vi "rio 9030.vi"() -> ()   [LabVIEW 2015]
uses:
  rio_Global.vi
  <vilib>/rvi/interface/nirviMethod/nirviMethod.xnode
  <vilib>/FPGAPlugInAG/Dynamic/niLvFpga_ReadFifo_Dynamic.vi
  <vilib>/rvi/errors/niLvFpgaMergeErrorWithErrorCode.vi
  <vilib>/FPGAPlugInAG/Dynamic/niLvFpga_Abort_Dynamic.vi
  <vilib>/FPGAPlugInAG/Dynamic/niLvFpga_Run_Dynamic.vi
  <vilib>/Analysis/Matrix/NI_Matrix.lvlib
  <vilib>/Analysis/Matrix/Numeric/Multiply/Multiply - RM,RM.vi
  <vilib>/Analysis/Matrix/Numeric/Subtract/Subtract - RM,RM.vi
  <vilib>/Analysis/Matrix/Numeric/Conversions/Array To Matrix - RA.vi
  <vilib>/Analysis/Matrix/Numeric/Add/Add - RM,RM.vi
  <vilib>/Analysis/NI_AALBase.lvlib
  <vilib>/rvi/interface/nirviReadWriteControl/nirviReadWriteControl.xnode
  <vilib>/Utility/error.llb/Error Cluster From Error Code.vi
  <vilib>/rvi/interface/Simulation/niFpgaSimulationCallBeginRW.vi
  <vilib>/rvi/errors/niLvFpgaAdjustHostInterfaceError.vi
  NiFpgaLv.dll
  <vilib>/rvi/interface/nirviOpenFPGA/nirviOpenFPGA.xnode
  FPGA Bitfiles/autonomous_FPGATarget4_fpga1_rudp+OsNkSQ.lvbitx
  samsung/fpga 1.vi
  <vilib>/Analysis/Matrix/Numeric/Multiply/Multiply - R,RM.vi
  <vilib>/Analysis/baseanly.llb/Real Inverse Matrix.vi
  <vilib>/Analysis/Matrix/Numeric/Conversions/Matrix To Array - RM.vi
  <vilib>/Analysis/Matrix/Numeric/Conversions/Array To Matrix - RA2.vi
panel:
  out "XY Graph":cluster{"Y":dbl[], "Y":dbl[]}[](graph)=[{"Y"=[1.82421875, 1.8301353427767753, 1.835194070339203, 1.8394013252854347, 1.8427635002136231, 1.84528698772192, 1.8469781804084777, 1.8478434708714486, 1.8478892517089844, 1.8471219155192375, 1.84554785490036, 1.8431734624505043, 1.8400051307678222, 1.8360492524504661, 1.8313122200965881, 1.8258004263043404, 1.819520263671875, 1.8124781247973443, 1.8046804022789003, 1.796133488714695, 1.7868437767028809, 1.77681765884161, 1.7660615277290344, 1.7545817759633064, 1.742384796142578, 1.7294769808650017, 1.7158647227287291, 1.701554414331913, 1.686552448272705, 1.6708652171492577, 1.654499113559723, 1.637460530102253, 1.619755859375, 1.6013914939761162, 1.5823738265037537, 1.5627092495560646, 1.5424041557312012, 1.5214649376273155, 1.4998979878425598, 1.4777096989750862, 1.4549064636230469, 1.431494674384594, 1.4074807238578795, 1.3828710046410562, 1.3576719093322753, 1.3318898305296898, 1.3055311608314515, 1.2786022928357124, 1.251109619140625, 1.2230595323443412], "Y"=[0.0, 0.5, 1.0, 1.5, 2.0, 2.5, 3.0, 3.5, 4.0, 4.5, 5.0, 5.5, 6.0, 6.5, 7.0, 7.5, 8.0, 8.5, 9.0, 9.5, 10.0, 10.5, 11.0, 11.5, 12.0, 12.5, 13.0, 13.5, 14.0, 14.5, 15.0, 15.5, 16.0, 16.5, 17.0, 17.5, 18.0, 18.5, 19.0, 19.5, 20.0, 20.5, 21.0, 21.5, 22.0, 22.5, 23.0, 23.5, 24.0, 24.5]}, {"Y"=[-1.22265625, -1.2167396572232247, -1.211680929660797, -1.2074736747145653, -1.2041114997863769, -1.20158801227808, -1.1998968195915223, -1.1990315291285514, -1.1989857482910156, -1.1997530844807625, -1.20132714509964, -1.2037015375494957, -1.2068698692321778, -1.2108257475495339, -1.2155627799034119, -1.2210745736956596, -1.227354736328125, -1.2343968752026557, -1.2421945977210997, -1.250741511285305, -1.2600312232971191, -1.27005734115839, -1.2808134722709656, -1.2922932240366936, -1.304490203857422, -1.3173980191349983, -1.3310102772712709, -1.345320585668087, -1.360322551727295, -1.3760097828507423, -1.392375886440277, -1.409414469897747, -1.427119140625, -1.4454835060238838, -1.4645011734962463, -1.4841657504439354, -1.5044708442687988, -1.5254100623726845, -1.5469770121574402, -1.5691653010249138, -1.5919685363769531, -1.615380325615406, -1.6393942761421205, -1.6640039953589438, -1.6892030906677247, -1.7149851694703102, -1.7413438391685485, -1.7682727071642876, -1.795765380859375, -1.8238154676556588, -1.8524165749549866, -1.8815623101592065, -1.911246280670166, -1.9414620938897134, -1.972203357219696, -2.003463678061962, -2.0352366638183597, -2.0675159218907355, -2.1002950596809384, -2.1335676845908162, -2.167327404022217, -2.2015678253769875, -2.2362825560569766, -2.2714652034640315, -2.307109375, -2.3432086780667305, -2.3797567200660703, -2.4167471083998677, -2.4541734504699706, -2.4920293536782263, -2.530308425426483, -2.5690042731165885, -2.6081105041503907, -2.647620725929737, -2.687528545856476, -2.7278275713324547, -2.7685114097595216, -2.809573668539524, -2.8510079550743104, -2.892807876765728, -2.934967041015625, -2.977479055225849, -3.020337526798248, -3.0635360631346704, -3.107068271636963, -3.150927759706974, -3.1951081347465515, -3.2396030041575434, -3.284405975341797, -3.3295106557011604, -3.3749106526374817, -3.4205995735526087, -3.466571025848389, -3.51281861692667, -3.5593359541893004], "Y"=[0.0, 0.5, 1.0, 1.5, 2.0, 2.5, 3.0, 3.5, 4.0, 4.5, 5.0, 5.5, 6.0, 6.5, 7.0, 7.5, 8.0, 8.5, 9.0, 9.5, 10.0, 10.5, 11.0, 11.5, 12.0, 12.5, 13.0, 13.5, 14.0, 14.5, 15.0, 15.5, 16.0, 16.5, 17.0, 17.5, 18.0, 18.5, 19.0, 19.5, 20.0, 20.5, 21.0, 21.5, 22.0, 22.5, 23.0, 23.5, 24.0, 24.5, 25.0, 25.5, 26.0, 26.5, 27.0, 27.5, 28.0, 28.5, 29.0, 29.5, 30.0, 30.5, 31.0, 31.5, 32.0, 32.5, 33.0, 33.5, 34.0, 34.5, 35.0, 35.5, 36.0, 36.5, 37.0, 37.5, 38.0, 38.5, 39.0, 39.5, 40.0, 40.5, 41.0, 41.5, 42.0, 42.5, 43.0, 43.5, 44.0, 44.5, 45.0, 45.5, 46.0, 46.5, 47.0]}, {"Y"=[-0.94, 0.94, 0.94, -0.94, -0.94], "Y"=[-3.2, -3.2, 1.5, 1.5, -3.2]}, {"Y"=[1.984375, 1.978057861328125, 1.9718017578125, 1.965606689453125, 1.95947265625], "Y"=[0.0, 0.5, 1.0, 1.5, 2.0]}, {"Y"=[-5.28125, -5.267578125, -5.25390625, -5.240234375, -5.2265625], "Y"=[0.0, 0.5, 1.0, 1.5, 2.0]}]
  out "x_view":dbl[](array[numeric])=[0.0, 0.5, 1.0, 1.5, 2.0, 2.5, 3.0, 3.5, 4.0, 4.5, 5.0, 5.5, 6.0, 6.5, 7.0, 7.5, 8.0, 8.5, 9.0, 9.5, 10.0, 10.5, 11.0, 11.5, 12.0, 12.5, 13.0, 13.5, 14.0, 14.5, 15.0, 15.5, 16.0, 16.5, 17.0, 17.5, 18.0, 18.5, 19.0, 19.5, 20.0, 20.5, 21.0, 21.5, 22.0, 22.5, 23.0, 23.5, 24.0, 24.5, 25.0, 25.5, 26.0, 26.5, 27.0, 27.5, 28.0, 28.5, 29.0, 29.5, 30.0, 30.5, 31.0, 31.5, 32.0, 32.5, 33.0, 33.5, 34.0, 34.5, 35.0, 35.5, 36.0, 36.5, 37.0, 37.5, 38.0, 38.5, 39.0, 39.5, 40.0, 40.5, 41.0, 41.5, 42.0, 42.5, 43.0, 43.5, 44.0, 44.5, 45.0, 45.5, 46.0, 46.5, 47.0, 47.5, 48.0, 48.5, 49.0, 49.5, 50.0, 50.5, 51.0, 51.5, 52.0, 52.5, 53.0, 53.5, 54.0, 54.5, 55.0, 55.5, 56.0, 56.5, 57.0, 57.5, 58.0, 58.5, 59.0, 59.5, 60.0, 60.5, 61.0, 61.5, 62.0, 62.5, 63.0, 63.5, 64.0, 64.5, 65.0, 65.5, 66.0, 66.5, 67.0, 67.5, 68.0, 68.5, 69.0, 69.5, 70.0, 70.5, 71.0, 71.5, 72.0, 72.5, 73.0, 73.5, 74.0, 74.5, 75.0, 75.5, 76.0, 76.5, 77.0, 77.5, 78.0, 78.5, 79.0, 79.5, 80.0, 80.5, 81.0, 81.5, 82.0, 82.5, 83.0, 83.5, 84.0, 84.5, 85.0, 85.5, 86.0, 86.5, 87.0, 87.5, 88.0, 88.5, 89.0, 89.5, 90.0, 90.5, 91.0, 91.5, 92.0, 92.5, 93.0, 93.5, 94.0, 94.5, 95.0, 95.5, 96.0, 96.5, 97.0, 97.5, 98.0, 98.5, 99.0, 99.5, 100.0, 100.5, 101.0, 101.5, 102.0, 102.5, 103.0, 103.5, 104.0, 104.5, 105.0, 105.5, 106.0, 106.5, 107.0, 107.5, 108.0, 108.5, 109.0, 109.5, 110.0, 110.5, 111.0, 111.5, 112.0, 112.5, 113.0, 113.5, 114.0, 114.5, 115.0, 115.5, 116.0, 116.5, 117.0, 117.5, 118.0, 118.5, 119.0, 119.5, 120.0, 120.5, 121.0, 121.5, 122.0, 122.5, 123.0, 123.5, 124.0, 124.5, 125.0, 125.5, 126.0, 126.5, 127.0, 127.5, 128.0]
  in  "rate limit":dbl=0.006 format="%#_13g"
  in  "Manual Steering torque":dbl(slide) min=-0.3 max=0.3 step=0.01 scale=-0.3..0.3
  out "T init":i32
  out "T out":i32
  out "PWM GAS":dbl=1000.0 min=1000.0 max=2000.0 step=1.0
  out "FPGA":refnum<k20>
  out "Mobileye_time 50":u32
  out "H_GPS":dbl
  out "vgain":dbl=1.0
  out "vcount":u64=1
  out "hbias":dbl
  out "hcount":u64=1
  out "get heading":bool
  out "get position":bool
  out "heading error":dbl
  out "h_gps":dbl
  out "rt":dbl
  out "pos error":dbl
  out "POS init":bool
  out "Heading":dbl
  out "pos":dbl[](array[numeric])
  in  "GPS init":bool=TRUE
  out "pos_gps":dbl[](array[numeric]) format="%#_19f"
  out "dt":dbl
  out "Pos_time 10":i32
  out "Ref_steer_planner":dbl
  out "Ref_vel_planner":dbl
  out "map":i32=2
  out "ecef ref":dbl[](array[numeric])
  in  "Velocity input":bool
  in  "manual Speed":dbl
  in  "Steer input":bool=TRUE
  out "Run":bool
  out "Auto":bool
  out "E - STOP":bool
  out "Con_time 10":i32
  out "VS_CAN":dbl
  out "CAN_time 10":u32
  out "gps1":refnum<visa-resource-name>
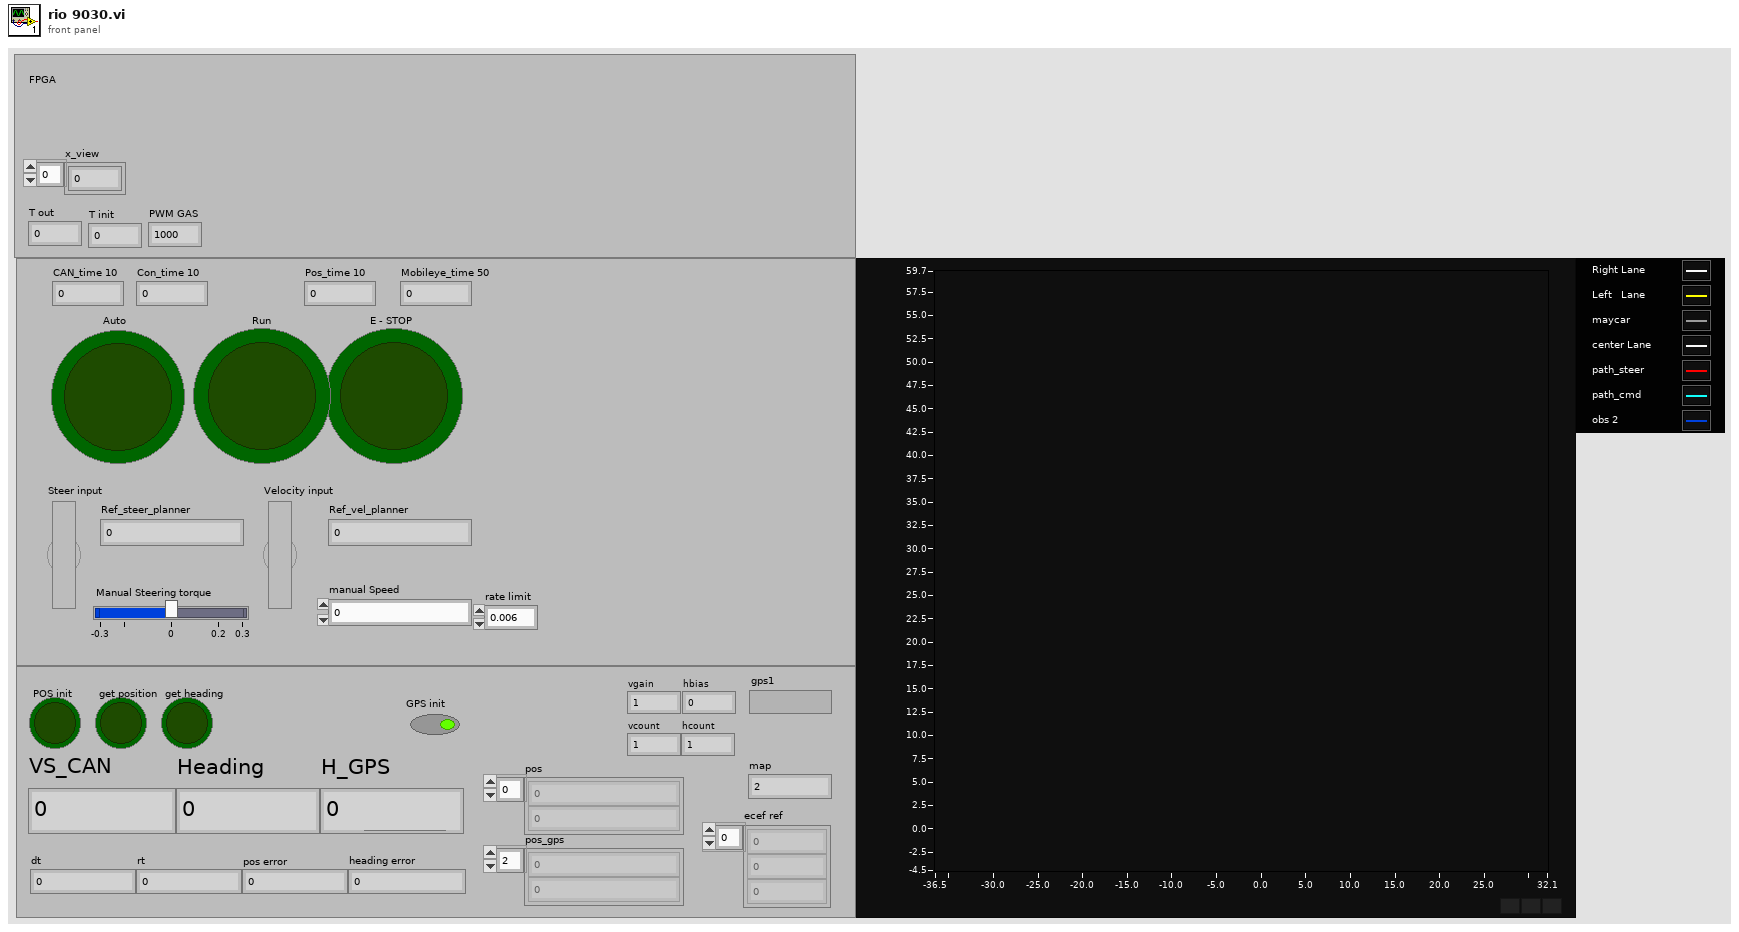
[diagram p1: front panel]
types:
  T1 = cluster{"identifier":u32, "timestamp":timestamp, "payload":u8[]}
  T2 = cluster{"connection ID":refnum<k16>, "net address":u32, "port":u16}
  T3 = cluster{"hash":i64, "sys time":i64, "mobileye time":u32, "ID":u32, "data":u8[]}
  T4 = cluster{"hash":i64, "sys time":i64, "car time":u32, "ID":u32, "data":u8[]}
  T5 = cluster{"hash":i64, "sys time":i64, "time":dbl, "yaw_rate":dbl, "mdps torque":dbl, "mdps str_ang":dbl, "VS_CAN":dbl, "lat_accel":dbl, "mcp":dbl, "accel pedal value":dbl, "tps":dbl, "odometer":dbl, "battery voltage":dbl, "WHL_SPD_RR":dbl, "WHL_SPD_RL":dbl, "WHL_SPD_FR":dbl, "WHL_SPD_FL":dbl}
  T6 = cluster{"hash":i64, "sys time":i64, "ref_vel":dbl, "ref_steer":dbl}
  T7 = cluster{"hash":i64, "sys time":i64, "time":dbl, "x":dbl, "y":dbl, "h":dbl, "numSV":i32, "postype":i32, "lag":i32, "hordev":dbl, "lat":dbl, "lon":dbl, "hgt":dbl, "map_idx":i32}
  T8 = cluster{"output[0]":dbl, "output[1]":dbl, "output[2]":dbl, "output[3]":dbl, "output[4]":dbl, "output[5]":dbl, "output[6]":dbl, "output[7]":dbl, "output[8]":dbl, "output[9]":dbl, "output[10]":dbl, "output[11]":dbl, "output[12]":dbl, "output[13]":dbl, "output[14]":dbl}
  T9 = cluster{"hash":i64, "sys time":i64, "time":dbl, "speed":dbl, "heading":dbl, "lat":dbl, "lon":dbl}
  T10 = cluster{"output[0]":dbl, "output[1]":dbl, "output[2]":dbl, "output[3]":dbl, "output[4]":dbl, "output[5]":dbl, "output[6]":dbl}
  T11 = typedef "NI_Matrix.lvlib/RealMatrix.ctl" = dbl[][]
  T12 = cluster{"hash":i64, "sys time":i64, "dt":dbl, "x":dbl, "y":dbl, "speed":dbl, "heading":dbl, "yaw_rate":dbl}
  T13 = cluster{"Real 2D Array[0]":dbl, "Real 2D Array[1]":dbl, "Real 2D Array[2]":dbl, "Real 2D Array[3]":dbl, "Real 2D Array[4]":dbl}
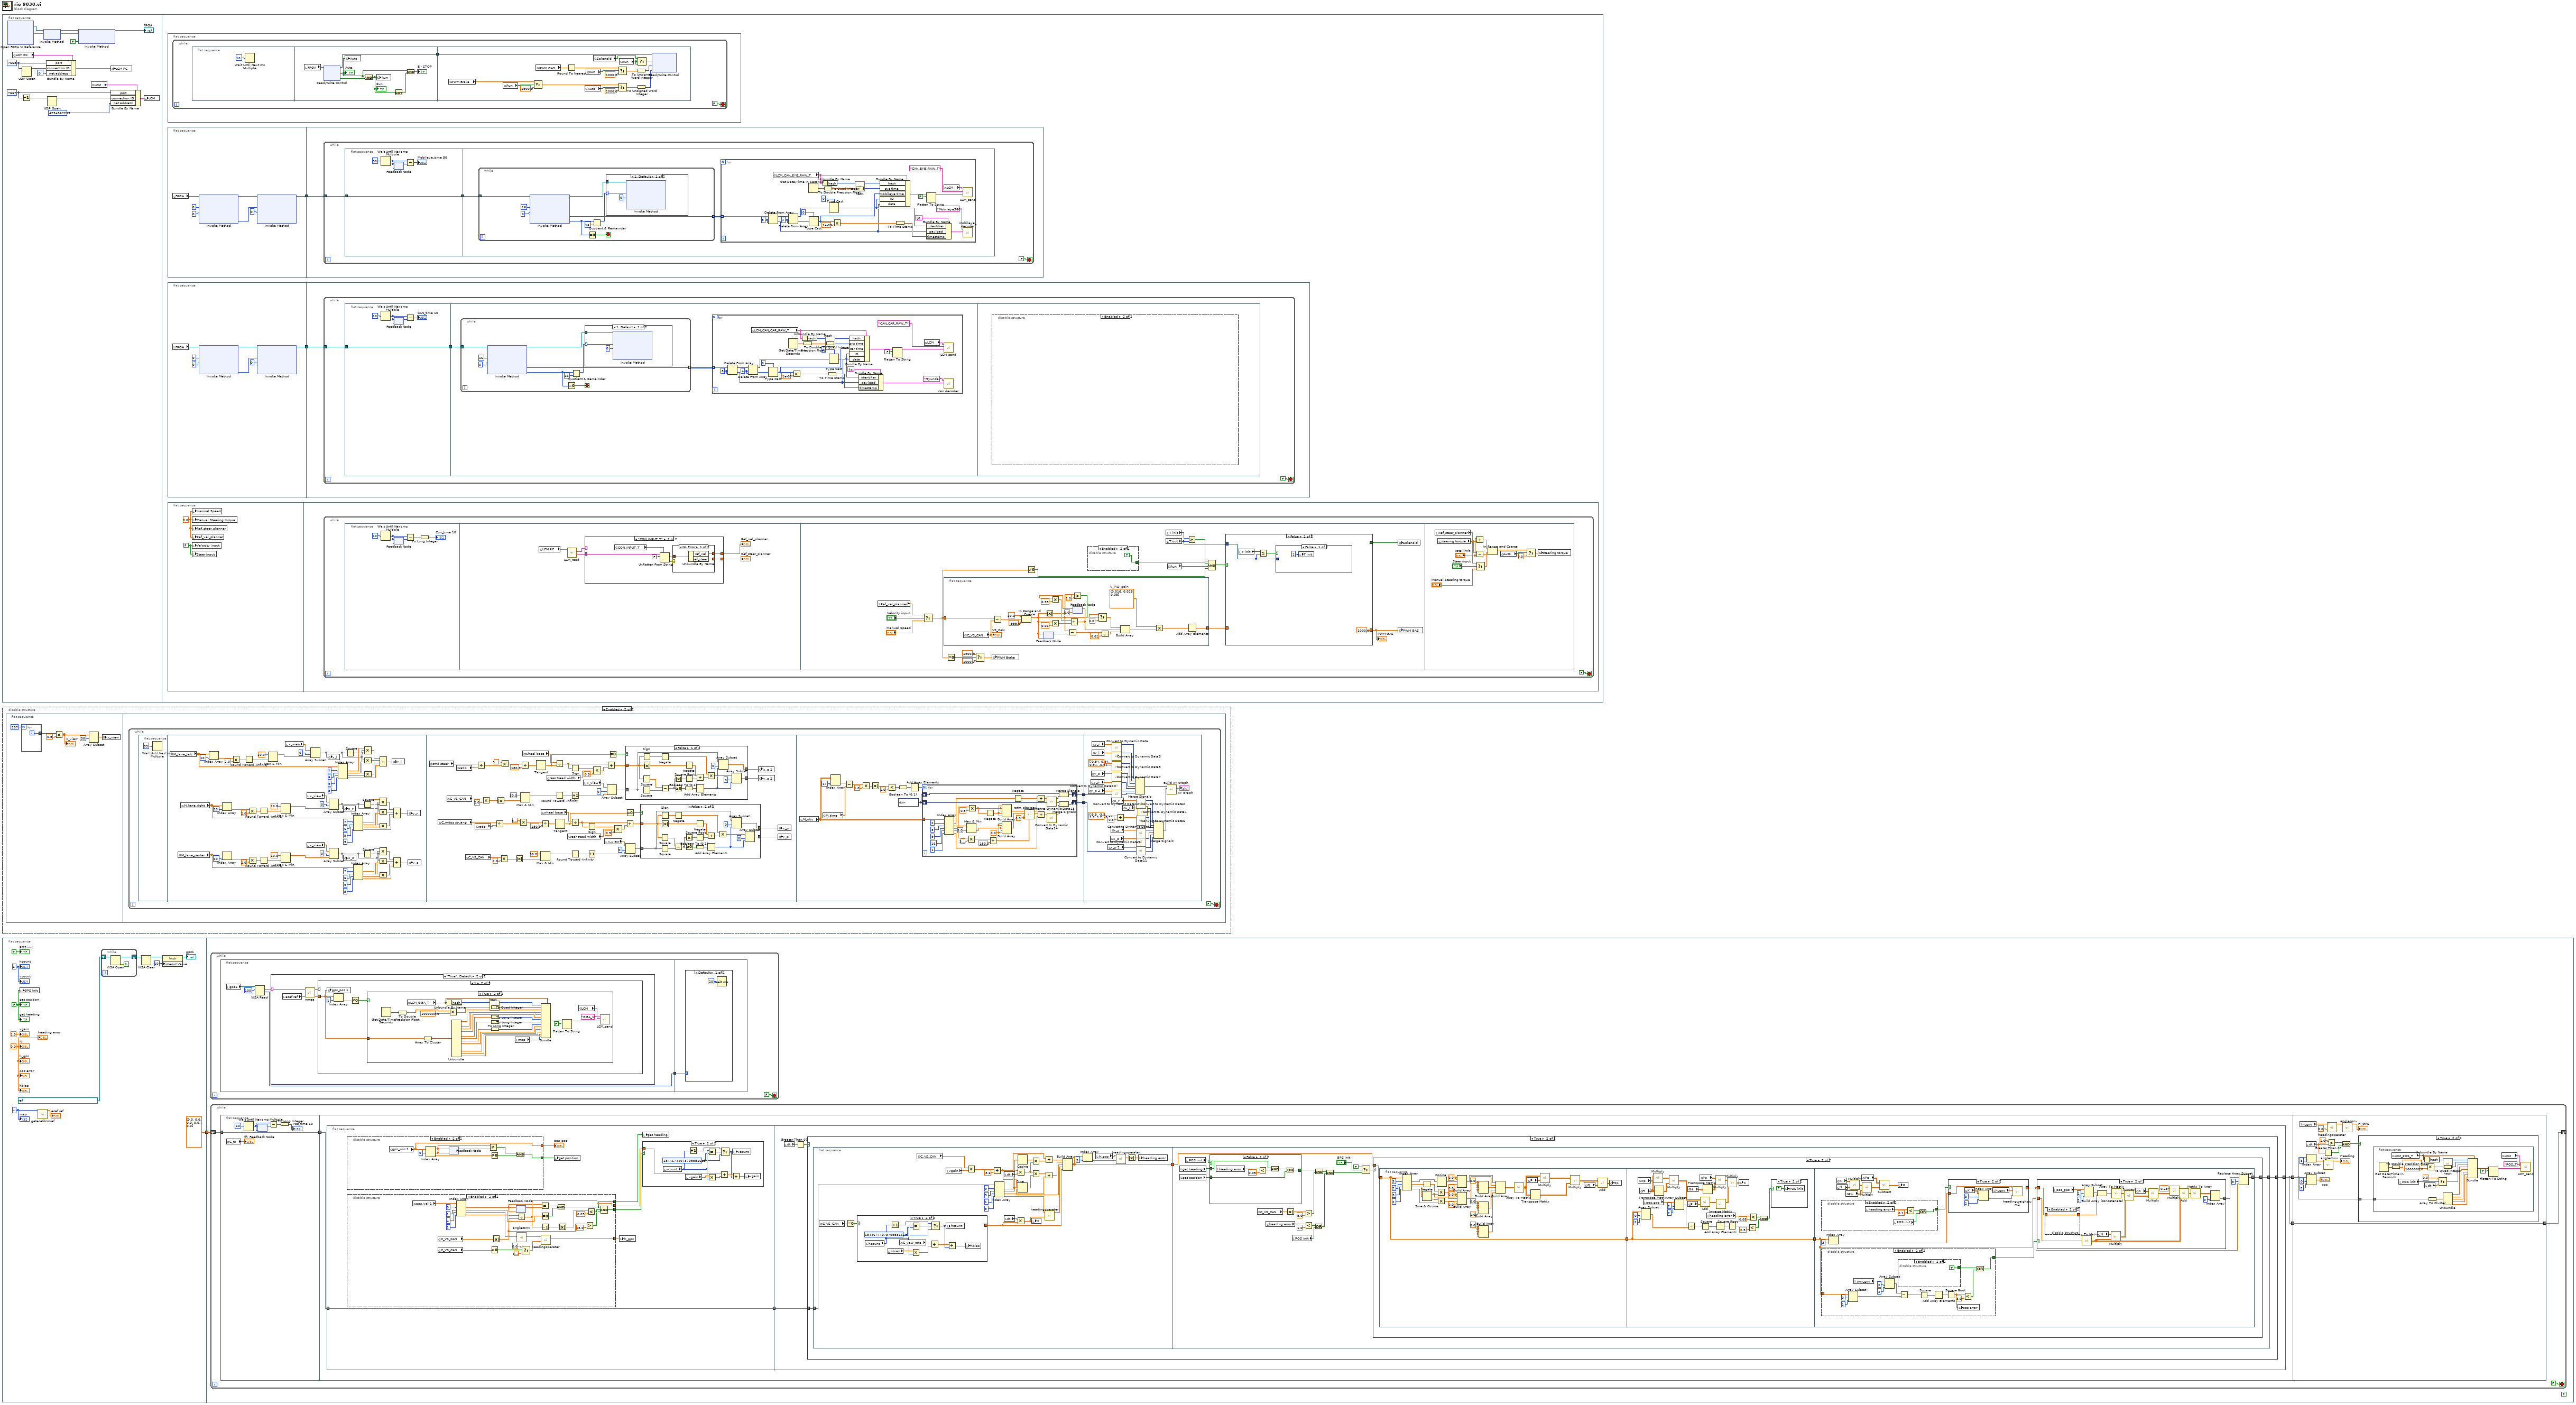
[diagram p0: block diagram]
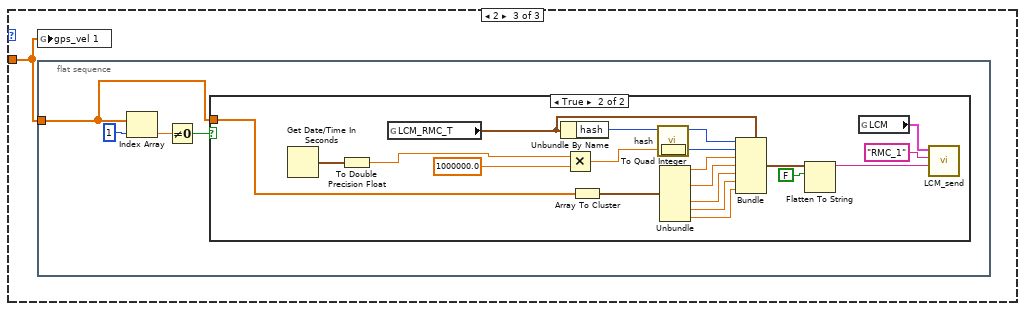
[diagram p5: hidden frame]
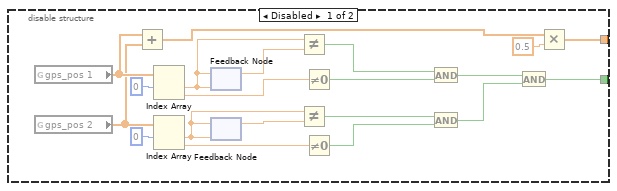
[diagram p8: hidden frame]
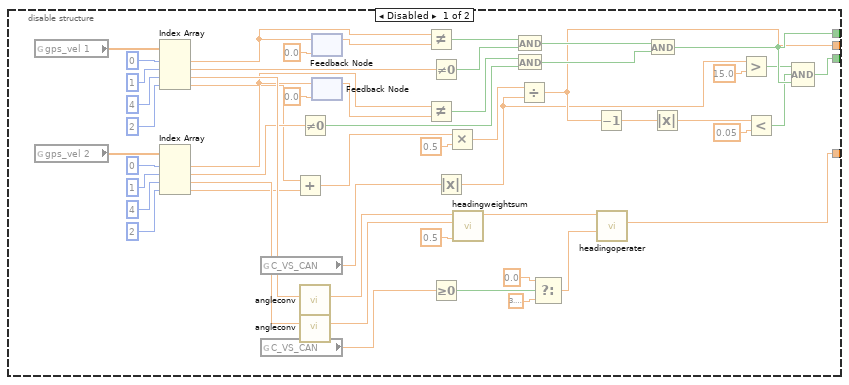
[diagram p9: hidden frame]
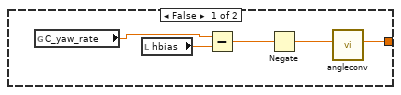
[diagram p12: hidden frame]
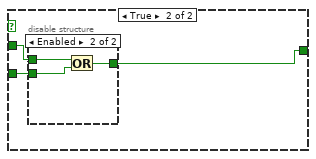
[diagram p13: hidden frame]
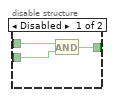
[diagram p14: hidden frame]
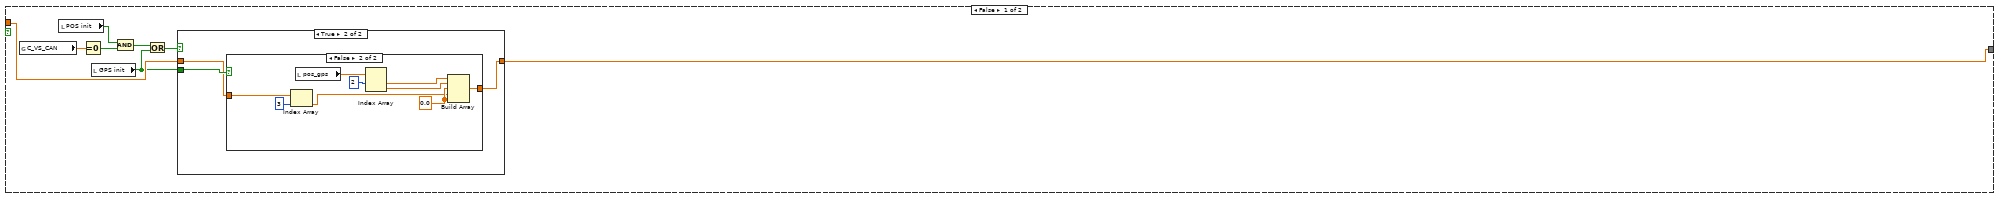
[diagram p15: hidden frame]
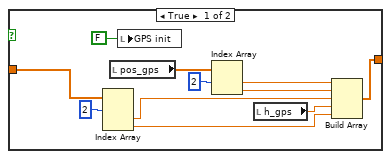
[diagram p17: hidden frame]
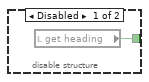
[diagram p19: hidden frame]
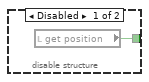
[diagram p20: hidden frame]
diagram:
  n1 = flat-sequence {
    frame #0 {
      w2 = u16 7668 ("port")
      w11 = u16 7667 ("port")
      n2 = xnode "Open FPGA VI Reference"() -> ("FPGA VI Reference Out"=w13:refnum<k20>, "error out"=w14:errorcluster)  [unwired: 2 in]
      n3 = global read "rio_Global.vi" "LCM PC"() -> (w6:T2)
      n4 = Decrement(x=w11) -> (x-1=w12:u16)
      n5 = UDP Open(11:w2) -> (port=w4:refnum<k16>)  [unwired: 4 in, 2 out]
      n6 = xnode "Invoke Method"("FPGA VI Reference In"=w13, "error in"=w14) -> ("FPGA VI Reference Out"=w15:refnum<k20>, "error out"=w16:errorcluster)
      n7 = Bundle By Name(cluster=w6, "port"=w2, "connection ID"=w4, "net address"=u32 0) -> (w5:T2)
      n8 = UDP Open(11:w12) -> (port=w9:refnum<k16>)  [unwired: 4 in, 2 out]
      n9 = xnode "Invoke Method"("FPGA VI Reference In"=w15, "error in"=w16, "Wait Until Done (F)"=FALSE) -> ("FPGA VI Reference Out"=→"FPGA":refnum<k20>)  [unwired: 1 out]
      n10 = global read "rio_Global.vi" "LCM"() -> (w7:T2)
      n11 = global write "rio_Global.vi" "LCM PC"(w5) -> ()
      n12 = Bundle By Name(cluster=w7, "port"=w11, "connection ID"=w9, "net address"=u32 4294967295) -> (w8:T2)
      n13 = global write "rio_Global.vi" "LCM"(w8) -> ()
    }
    frame #1 {
      n14 = flat-sequence {
        frame #0 {
          n15 = while {
            stop <- FALSE stop-if-true
            n16 = flat-sequence {
              tunnel: [w129] -> w126
              tunnel: w126 -> [w153]
              frame #0 {
                n17 = Wait Until Next ms Multiple(millisecond multiple=u32 10) -> ()  [unwired: 1 out]
              }
              frame #1 {
                n18 = local read "FPGA"() -> (w135:refnum<k20>)
                n19 = xnode "Read/Write Control"("FPGA VI Reference In"=w135) -> ("FPGA VI Reference Out"=w129:refnum<k20>, "Auto"=w131:bool, "Run"=w134:bool)  [unwired: 1 in, 1 out]
                "Auto" <- w131
                n20 = global write "rio_Global.vi" "Auto"(w131) -> ()
                n21 = And(x=w131, y=w134) -> (x .and. y?=w132:bool)
                "Run" <- w132
                n22 = global write "rio_Global.vi" "Run"(w132) -> ()
                n23 = Not(x=w132) -> (.not. x?=w130:bool)
                n24 = And(x=w131, y=w130) -> (x .and. y?=→"E - STOP":bool)
              }
              frame #2 {
                n25 = global read "rio_Global.vi" "PWM Brake"() -> (w139:dbl)
                n26 = global read "rio_Global.vi" "Run"() -> (w144:bool)
                n27 = Select(t=w139, s=w144, f=1900.0 ("t")) -> (s? t:f=w143:dbl)
                n28 = global read "rio_Global.vi" "PWM GAS"() -> (w152:dbl)
                n29 = Round To Nearest(number=w152) -> (nearest integer value=w141:dbl)
                n30 = global read "rio_Global.vi" "Auto"() -> (w147:bool)
                n31 = global read "rio_Global.vi" "Run"() -> (w149:bool)
                n32 = global read "rio_Global.vi" "Solenoid"() -> (w140:bool)
                n33 = Select(t=w141, s=w149, f=1000.0) -> (s? t:f=w137:dbl)
                n34 = Select(t=w143, s=w147, f=1000.0) -> (s? t:f=w138:dbl)
                n35 = global read "rio_Global.vi" "Run"() -> (w150:bool)
                n36 = To Unsigned Word Integer(number=w137) -> (unsigned 16bit integer=w148:u16)
                n37 = To Unsigned Word Integer(number=w138) -> (unsigned 16bit integer=w145:u16)
                n38 = Select(t=w140, s=w150, f=w150) -> (s? t:f=w136:bool)
                n39 = xnode "Read/Write Control"("FPGA VI Reference In"=w153, "Solenoid"=w136, "PWM Gas"=w148, "PWM Brake"=w145) -> ()  [unwired: 1 in, 2 out]
              }
            }
          }
        }
      }
      n40 = flat-sequence {
        tunnel: [w154] -> w19
        tunnel: w19 -> [w161]
        frame #0 {
          n41 = local read "FPGA"() -> (w155:refnum<k20>)
          n42 = xnode "Invoke Method"("FPGA VI Reference In"=w155, "Number of Elements"=u32 0, "Timeout (ms)"=0) -> ("FPGA VI Reference Out"=w157:refnum<k20>, "Elements Remaining"=w158:u32)  [unwired: 1 in, 2 out]
          n43 = xnode "Invoke Method"("FPGA VI Reference In"=w157, "Number of Elements"=w158, "Timeout (ms)"=0) -> ("FPGA VI Reference Out"=w154:refnum<k20>)  [unwired: 1 in, 3 out]
        }
        frame #1 {
          n44 = while {
            tunnel: w161 -> [w162]
            stop <- FALSE stop-if-true
            n45 = flat-sequence {
              tunnel: [w165] -> w163
              tunnel: w162 -> [w165]
              tunnel: w163 -> [w171]
              frame #0 {
                n46 = Wait Until Next ms Multiple(millisecond multiple=u32 50) -> (millisecond timer value=w167:u32)
                n47 = feedback #1(w167) -> (w168:u32)
                n48 = feedback-in #1(w167) -> ()
                n49 = Subtract(x=w167, y=w168) -> (x-y=→"Mobileye_time 50":u32)
              }
              frame #1 {
                n50 = while {
                  tunnel: w171 -> [w208]
                  tunnel: [w205] -> w170 mode=indexing
                  stop <- w203 stop-if-true
                  n51 = xnode "Invoke Method"("FPGA VI Reference In"=w208, "Number of Elements"=u32 16, "Timeout (ms)"=0) -> ("FPGA VI Reference Out"=w204:refnum<k20>, "Data"=w205:u8[], "Elements Remaining"=w202:u32)  [unwired: 1 in, 1 out]
                  n52 = Equal To 0?(x=w202) -> (x = 0?=w203:bool)
                  n53 = Quotient & Remainder(x=w202, y=u32 16) -> (x-y*floor(x/y)=w200:u32)  [unwired: 1 out]
                  n54 = case shown="1, Default" w200 {
                    selector: w200 -> [w211 _]
                    tunnel: w204 -> [w210 _]
                    frame 1, Default {
                      n55 = xnode "Invoke Method"("FPGA VI Reference In"=w210, "Number of Elements"=w211, "Timeout (ms)"=0) -> ()  [unwired: 1 in, 4 out]
                    }
                    frame 0 {
                    }
                  }
                }
                n56 = for {
                  tunnel: w170 -> [w192] mode=indexing
                  w195 = 4 ("length")
                  w193 = 8 ("index")
                  n57 = Delete From Array(array=w192, length=w193, index=w193) -> (deleted portion=w172:u8[], array with subset deleted=w194:u8[])
                  n58 = global read "rio_Global.vi" "LCM_CAN_EYE_RAW_T"() -> (w180:T3)
                  n59 = Delete From Array(array=w194, length=w195, index=w195) -> (deleted portion=w199:u8[], array with subset deleted=w196:u8[])
                  n60 = Get Date/Time In Seconds() -> (seconds since 1Jan1904=w183:timestamp)
                  n61 = Type Cast(type=u32 0, x=w199) -> (*(type *) &x=w174:u32)
                  n62 = Unbundle By Name(w180) -> ("hash"=w181:i64)
                  n63 = To Double Precision Float(number=w183) -> (double precision float=w184:dbl)
                  n64 = Type Cast(type=u32 0, x=w196) -> (*(type *) &x=w173:u32)
                  n65 = Multiply(x=w174, y=1e-07) -> (x*y=w190:dbl)
                  n66 = call "hash.vi"("input"=w181) -> ("output"=w179:i64)  [unwired: 10 in]
                  n67 = To Quad Integer(1:w184) -> (0:w185:i64)
                  n68 = Bundle By Name(cluster=w180, "hash"=w179, "sys time"=w185, "mobileye time"=w174, "ID"=w173, "data"=w172) -> (w177:T3)
                  n69 = To Time Stamp(1:w190) -> (0:w188:timestamp)
                  n70 = Flatten To String(anything=w177, prepend array or string size? (T)=FALSE) -> (data string=w175:string)  [unwired: 2 in, 2 out]
                  n71 = Bundle By Name(cluster=T1 {"identifier"=0, "timestamp"=timestamp(0 s since 1904-01-01), "payload"=[]} ("can cluster"), "identifier"=w173, "payload"=w172, "timestamp"=w188) -> (w186:T1)
                  n72 = global read "rio_Global.vi" "LCM"() -> (w176:T2)
                  n73 = call "LCM_send.vi"("DATA"=w175, "ID"="CAN_EYE_RAW_T", "LCM"=w176) -> ()  [unwired: 6 in, 3 out]
                  n74 = call "mobileye_decoder.vi"("can cluster"=w186, "name"="Mobileye560") -> ()  [unwired: 10 in]
                }
              }
            }
          }
        }
      }
      n75 = flat-sequence {
        tunnel: [w212] -> w20
        tunnel: w20 -> [w219]
        frame #0 {
          n76 = local read "FPGA"() -> (w213:refnum<k20>)
          n77 = xnode "Invoke Method"("FPGA VI Reference In"=w213, "Number of Elements"=u32 0, "Timeout (ms)"=0) -> ("FPGA VI Reference Out"=w215:refnum<k20>, "Elements Remaining"=w214:u32)  [unwired: 1 in, 2 out]
          n78 = xnode "Invoke Method"("FPGA VI Reference In"=w215, "Number of Elements"=w214, "Timeout (ms)"=0) -> ("FPGA VI Reference Out"=w212:refnum<k20>)  [unwired: 1 in, 3 out]
        }
        frame #1 {
          n79 = while {
            tunnel: w219 -> [w220]
            stop <- FALSE stop-if-true
            n80 = flat-sequence {
              tunnel: [w223] -> w221
              tunnel: w220 -> [w223]
              tunnel: w221 -> [w228]
              frame #0 {
                n81 = Wait Until Next ms Multiple(millisecond multiple=u32 10) -> (millisecond timer value=w226:u32)
                n82 = feedback #2(w226) -> (w225:u32)
                n83 = feedback-in #2(w226) -> ()
                n84 = Subtract(x=w226, y=w225) -> (x-y=→"CAN_time 10":u32)
              }
              frame #1 {
                n85 = while {
                  tunnel: w228 -> [w238]
                  tunnel: [w235] -> w229 mode=indexing
                  stop <- w234 stop-if-true
                  n86 = xnode "Invoke Method"("FPGA VI Reference In"=w238, "Number of Elements"=u32 16, "Timeout (ms)"=0) -> ("FPGA VI Reference Out"=w233:refnum<k20>, "Data"=w235:u8[], "Elements Remaining"=w230:u32)  [unwired: 1 in, 1 out]
                  n87 = Equal To 0?(x=w230) -> (x = 0?=w234:bool)
                  n88 = Quotient & Remainder(x=w230, y=u32 16) -> (x-y*floor(x/y)=w231:u32)  [unwired: 1 out]
                  n89 = case shown="1, Default" w231 {
                    selector: w231 -> [w241 _]
                    tunnel: w233 -> [w240 _]
                    frame 1, Default {
                      n90 = xnode "Invoke Method"("FPGA VI Reference In"=w240, "Number of Elements"=w241, "Timeout (ms)"=0) -> ()  [unwired: 1 in, 4 out]
                    }
                    frame 0 {
                    }
                  }
                }
                n91 = for {
                  tunnel: w229 -> [w262] mode=indexing
                  w265 = 4 ("length")
                  w263 = 8 ("index")
                  n92 = Delete From Array(array=w262, length=w263, index=w263) -> (deleted portion=w245:u8[], array with subset deleted=w264:u8[])
                  n93 = Delete From Array(array=w264, length=w265, index=w265) -> (deleted portion=w269:u8[], array with subset deleted=w266:u8[])
                  n94 = global read "rio_Global.vi" "LCM_CAN_CAR_RAW_T"() -> (w250:T4)
                  n95 = Type Cast(type=u32 0, x=w269) -> (*(type *) &x=w247:u32)
                  n96 = Get Date/Time In Seconds() -> (seconds since 1Jan1904=w244:timestamp)
                  n97 = Multiply(x=w247, y=1e-07) -> (x*y=w258:dbl)
                  n98 = Unbundle By Name(w250) -> ("hash"=w249:i64)
                  n99 = To Double Precision Float(number=w244) -> (double precision float=w243:dbl)
                  n100 = call "hash.vi"("input"=w249) -> ("output"=w251:i64)  [unwired: 10 in]
                  n101 = To Quad Integer(1:w243) -> (0:w242:i64)
                  n102 = To Time Stamp(1:w258) -> (0:w257:timestamp)
                  n103 = Type Cast(type=u32 0, x=w266) -> (*(type *) &x=w246:u32)
                  n104 = Bundle By Name(cluster=w250, "hash"=w251, "sys time"=w242, "car time"=w247, "ID"=w246, "data"=w245) -> (w253:T4)
                  n105 = Bundle By Name(cluster=T1 {"identifier"=0, "timestamp"=timestamp(0 s since 1904-01-01), "payload"=[]} ("can cluster"), "identifier"=w246, "payload"=w245, "timestamp"=w257) -> (w260:T1)
                  n106 = Flatten To String(anything=w253, prepend array or string size? (T)=FALSE) -> (data string=w255:string)  [unwired: 2 in, 2 out]
                  n107 = global read "rio_Global.vi" "LCM"() -> (w254:T2)
                  n108 = call "LCM_send.vi"("DATA"=w255, "ID"="CAN_CAR_RAW_T", "LCM"=w254) -> ()  [unwired: 6 in, 3 out]
                  n109 = call "can decoder.vi"("can cluster"=w260, "name"="Hyundai" ("vehicle name")) -> ()  [unwired: 10 in]
                }
              }
              frame #2 {
                n110 = disable-structure shown="Enabled" {
                  frame Disabled {
                    n111 = Get Date/Time In Seconds() -> (seconds since 1Jan1904=w280:timestamp)
                    n112 = To Double Precision Float(number=w280) -> (double precision float=w279:dbl)
                    n113 = global read "rio_Global.vi" "LCM_CAN_T"() -> (w297:T5)
                    n114 = global read "rio_Global.vi" "C_MCP"() -> (w298:dbl)
                    n115 = Unbundle By Name(w297) -> ("hash"=w296:i64)
                    n116 = global read "rio_Global.vi" "time"() -> (w299:dbl)
                    n117 = Multiply(x=w279, y=1000000.0) -> (x*y=w277:dbl)
                    n118 = global read "rio_Global.vi" "C_battery voltage"() -> (w286:dbl)
                    n119 = global read "rio_Global.vi" "C_mdps str_ang"() -> (w291:dbl)
                    n120 = global read "rio_Global.vi" "C_WHL_SPD_RR"() -> (w275:dbl)
                    n121 = global read "rio_Global.vi" "C_WHL_SPD_RL"() -> (w274:dbl)
                    n122 = global read "rio_Global.vi" "C_WHL_SPD_FR"() -> (w273:dbl)
                    n123 = global read "rio_Global.vi" "C_mdps torque"() -> (w292:dbl)
                    n124 = global read "rio_Global.vi" "C_WHL_SPD_FL"() -> (w272:dbl)
                    n125 = global read "rio_Global.vi" "C_odometer"() -> (w284:dbl)
                    n126 = global read "rio_Global.vi" "C_yaw_rate"() -> (w293:dbl)
                    n127 = global read "rio_Global.vi" "C_lat_accel"() -> (w290:dbl)
                    n128 = global read "rio_Global.vi" "C_VS_CAN"() -> (w285:dbl)
                    n129 = global read "rio_Global.vi" "C_APV"() -> (w287:dbl)
                    n130 = call "hash.vi"("input"=w296) -> ("output"=w295:i64)  [unwired: 10 in]
                    n131 = To Quad Integer(1:w277) -> (0:w276:i64)
                    n132 = To Double Precision Float(number=w299) -> (double precision float=w294:dbl)
                    n133 = To Double Precision Float(number=w298) -> (double precision float=w289:dbl)
                    n134 = global read "rio_Global.vi" "C_tps"() -> (w288:dbl)
                    n135 = Bundle By Name(cluster=w297, "hash"=w295, "sys time"=w276, "time"=w294, "yaw_rate"=w293, "mdps torque"=w292, "mdps str_ang"=w291, "VS_CAN"=w285, "lat_accel"=w290, "mcp"=w289, "accel pedal value"=w287, "tps"=w288, "odometer"=w284, "battery voltage"=w286, "WHL_SPD_RR"=w275, "WHL_SPD_RL"=w274, "WHL_SPD_FR"=w273, "WHL_SPD_FL"=w272) -> (w283:T5)
                    n136 = Flatten To String(anything=w283, prepend array or string size? (T)=FALSE) -> (data string=w282:string)  [unwired: 2 in, 2 out]
                    n137 = global read "rio_Global.vi" "LCM"() -> (w271:T2)
                    n138 = call "LCM_send.vi"("DATA"=w282, "ID"="CAN_T", "LCM"=w271) -> ()  [unwired: 6 in, 3 out]
                  }
                  frame Enabled {
                  }
                }
              }
            }
          }
        }
      }
      n139 = flat-sequence {
        frame #0 {
          w22 = 0.0 ("Ref_vel_planner")
          w21 = FALSE ("GPS init")
          n140 = local write "manual Speed"(w22) -> ()
          n141 = local write "Manual Steering torque"(w22) -> ()
          n142 = local write "Ref_steer_planner"(w22) -> ()
          n143 = local write "Ref_vel_planner"(w22) -> ()
          n144 = local write "Velocity input"(w21) -> ()
          n145 = local write "Steer input"(w21) -> ()
        }
        frame #1 {
          n146 = while {
            stop <- FALSE stop-if-true
            n147 = flat-sequence {
              frame #0 {
                n148 = Wait Until Next ms Multiple(millisecond multiple=u32 10) -> (millisecond timer value=w27:u32)
                n149 = feedback #3(w27) -> (w26:u32)
                n150 = feedback-in #3(w27) -> ()
                n151 = Subtract(x=w27, y=w26) -> (x-y=w25:u32)
                n152 = To Long Integer(number=w25) -> (32bit integer=→"Con_time 10":i32)
              }
              frame #1 {
                n153 = global read "rio_Global.vi" "LCM PC"() -> (w33:T2)
                n154 = call "LCM_read.vi"("LCM"=w33) -> ("data"=w31:string, "ID"=w32:string)  [unwired: 7 in, 2 out]
                n155 = case shown="\"CON_INPUT_T\"" w32 {
                  tunnel: w31 -> [_ w36]
                  tunnel: [_ w35] -> w30
                  tunnel: [_ w34] -> w29
                  frame "False", Default {
                  }
                  frame "CON_INPUT_T" {
                    n156 = global read "rio_Global.vi" "CON_INPUT_T"() -> (w38:T6)
                    n157 = Unflatten From String(type=w38, binary string=w36, data includes array or string size? (T)=FALSE) -> (value=w37:T6, error out=w39:errorcluster)  [unwired: 2 in, 1 out]
                    n158 = case shown="No Error" w39 {
                      tunnel: w37 -> [w43 _]
                      tunnel: [w42 _] -> w35
                      tunnel: [w41 _] -> w34
                      frame No Error {
                        n159 = Unbundle By Name(w43) -> ("ref_vel"=w42:dbl, "ref_steer"=w41:dbl)
                      }
                      frame Error {
                      }
                    }
                  }
                }
                "Ref_vel_planner" <- w30
                "Ref_steer_planner" <- w29
              }
              frame #2 {
                n160 = local read "Ref_vel_planner"() -> (w59:dbl)
                n161 = Select(t=w59, s="Velocity input", f="manual Speed") -> (s? t:f=w48:dbl)
                n162 = flat-sequence {
                  tunnel: w48 -> [w112]
                  tunnel: [w111] -> w51
                  frame #0 {
                    w94 = dbl[] [0.016, 0.025, 0.08]  # V_PID_gain
                    n163 = global read "rio_Global.vi" "C_VS_CAN"() -> (w88:dbl)
                    "VS_CAN" <- w88
                    n164 = Subtract(x=w112, y=w88) -> (x-y=w113:dbl)
                    n165 = In Range and Coerce(upper limit=20.0, x=w113, lower limit=-999.0) -> (coerced(x)=w90:dbl)  [unwired: 1 out]
                    n166 = feedback #4(w90) -> (w92:dbl)
                    n167 = feedback-in #4(w90) -> ()
                    n168 = Absolute Value(x=w90) -> (abs(x)=w98:dbl)
                    n169 = Multiply(x=w90, y=0.01) -> (x*y=w108:dbl)
                    n170 = Subtract(x=w90, y=w92) -> (x-y=w91:dbl)
                    n171 = Greater?(x=w98, y=1.0) -> (0:w95:bool)
                    n172 = feedback #5(0.0) -> (w107:dbl)
                    n173 = Multiply(x=w107, y=0.95) -> (x*y=w101:dbl)
                    n174 = Add(x=w101, y=w108) -> (x+y=w102:dbl)
                    n175 = feedback-in #5(w102) -> ()
                    n176 = Select(t=w90, s=w95, f=0.0) -> (s? t:f=w105:dbl)
                    n177 = Divide(x=w91, y=0.01) -> (x/y=w89:dbl)
                    n178 = Build Array(w105, w102, w89) -> (w104:dbl[])
                    n179 = Multiply(x=w94, y=w104) -> (x*y=w103:dbl[])
                    n180 = Add Array Elements(numeric array=w103) -> (sum=w111:dbl)
                  }
                }
                n181 = Equal To 0?(x=w48) -> (x = 0?=w47:bool)
                n182 = Select(t=1900.0, s=w47, f=1000.0) -> (s? t:f=w46:dbl)
                n183 = global write "rio_Global.vi" "PWM Brake"(w46) -> ()
                n184 = Not Equal To 0?(x=w48) -> (x != 0?=w56:bool)
                n185 = disable-structure shown="Enabled" {
                  disable-tunnel: [w64 TRUE] -> w52
                  frame Disabled {
                    n186 = global read "rio_Global.vi" "C_MCP"() -> (w63:dbl)
                    n187 = Less?(x=w63, y=5.0) -> (x < y?=w64:bool)
                  }
                  frame Enabled {
                  }
                }
                n188 = local read "T init"() -> (w55:i32)
                n189 = local read "T out"() -> (w54:i32)
                n190 = global read "rio_Global.vi" "Run"() -> (w50:bool)
                n191 = Greater Or Equal?(x=w55, y=w54) -> (x >= y?=w49:bool)
                n192 = Compound Arithmetic op=AND(w49, w52, w50, w56) -> (w53:bool)
                n193 = case shown="False" w53 {
                  tunnel: [1000.0 ("Numeric") w80] -> w57
                  tunnel: w51 -> [_ w82]
                  tunnel: w54 -> [w66 _]
                  tunnel: [_ TRUE] -> w58
                  frame False {
                    n194 = local read "T init"() -> (w67:i32)
                    n195 = Less Or Equal?(x=w67, y=w66) -> (x <= y?=w68:bool)
                    n196 = case shown="False" w68 {
                      tunnel: w66 -> [_ w71]
                      frame False {
                        n197 = local write "T init"(1 ("T init")) -> ()
                      }
                      frame True {
                        n198 = local read "T init"() -> (w74:i32)
                        n199 = Increment(x=w74) -> (x+1=w73:i32)
                        n200 = Max & Min(x=w73, y=w71) -> (min(x,y)=w72:i32)  [unwired: 1 out]
                        n201 = local write "T init"(w72) -> ()
                      }
                    }
                  }
                  frame True {
                    n202 = To Long Integer(number=w82) -> (32bit integer=w84:i32)
                    n203 = Multiply(x=10.0, y=w82) -> (x*y=w79:dbl)
                    n204 = global read "rio_Global.vi" "PWM GAS"() -> (w75:dbl)
                    n205 = Add(x=w84, y=20) -> (x+y=w86:i32)
                    "T out" <- w86
                    n206 = Add(x=w79, y=w75) -> (x+y=w77:dbl)
                    n207 = Increment(x=w86) -> (x+1=→"T init":i32)
                    n208 = In Range and Coerce(upper limit=1700.0, x=w77, lower limit=1000.0 ("x")) -> (coerced(x)=w80:dbl)  [unwired: 1 out]
                  }
                }
                "PWM GAS" <- w57
                n209 = global write "rio_Global.vi" "Solenoid"(w58) -> ()
                n210 = global write "rio_Global.vi" "PWM GAS"(w57) -> ()
              }
              frame #3 {
                n211 = local read "Ref_steer_planner"() -> (w125:dbl)
                n212 = global read "rio_Global.vi" "steering torque"() -> (w123:dbl)
                n213 = Add(x="rate limit", y=w123) -> (x+y=w121:dbl)
                n214 = Subtract(x=w123, y="rate limit") -> (x-y=w119:dbl)
                n215 = Select(t=w125, s="Steer input", f="Manual Steering torque") -> (s? t:f=w120:dbl)
                n216 = In Range and Coerce(upper limit=w121, x=w120, lower limit=w119) -> (coerced(x)=w117:dbl)  [unwired: 1 out]
                n217 = global read "rio_Global.vi" "Auto"() -> (w116:bool)
                n218 = Select(t=w117, s=w116, f=0.0) -> (s? t:f=w115:dbl)
                n219 = global write "rio_Global.vi" "steering torque"(w115) -> ()
              }
            }
          }
        }
      }
    }
  }
  n220 = disable-structure shown="Enabled" {
    frame Disabled {
    }
    frame Enabled {
      n221 = flat-sequence {
        frame #0 {
          n222 = for {
            N: 257 -> [_]
            tunnel: [w306] -> w304 mode=indexing
            i -> [w306]
          }
          n223 = Multiply(x=w304, y=0.5) -> (x*y=w302:dbl[])
          "x_view" <- w302
          n224 = Array Subset(array=w302, index=30) -> (w300:dbl[])  [unwired: 1 in]
          n225 = global write "rio_Global.vi" "x_view"(w300) -> ()
        }
        frame #1 {
          n226 = while {
            stop <- FALSE stop-if-true
            n227 = flat-sequence {
              tunnel: [w490] -> w308
              tunnel: [w489] -> w307
              tunnel: w308 -> [w548]
              tunnel: w307 -> [w550]
              frame #0 {
                n228 = Wait Until Next ms Multiple(millisecond multiple=u32 33) -> ()  [unwired: 1 out]
              }
              frame #1 {
                n229 = global read "rio_Global.vi" "M_lane_left"() -> (w317:dbl[])
                n230 = global read "rio_Global.vi" "M_lane_center"() -> (w319:dbl[])
                n231 = global read "rio_Global.vi" "M_lane_right"() -> (w318:dbl[])
                n232 = Index Array(array=w317, index=10) -> (element=w348:dbl)
                n233 = Index Array(array=w318, index=10) -> (element=w357:dbl)
                n234 = Index Array(array=w319, index=10) -> (element=w326:dbl)
                n235 = Multiply(x=w348, y=2.0) -> (x*y=w349:dbl)
                n236 = Round Toward -Infinity(1:w349) -> (0:w342:dbl)
                n237 = Multiply(x=w357, y=2.0) -> (x*y=w356:dbl)
                n238 = Multiply(x=w326, y=2.0) -> (x*y=w337:dbl)
                n239 = Round Toward -Infinity(1:w356) -> (0:w346:dbl)
                n240 = Round Toward -Infinity(1:w337) -> (0:w322:dbl)
                n241 = Max & Min(x=10.0, y=w342) -> (max(x,y)=w341:dbl)  [unwired: 1 out]
                n242 = Max & Min(x=10.0, y=w346) -> (max(x,y)=w344:dbl)  [unwired: 1 out]
                n243 = Max & Min(x=10.0, y=w322) -> (max(x,y)=w340:dbl)  [unwired: 1 out]
                n244 = local read "x_view"() -> (w350:dbl[])
                n245 = local read "x_view"() -> (w355:dbl[])
                n246 = local read "x_view"() -> (w325:dbl[])
                n247 = Array Subset(array=w350, index=0, length=w341) -> (w311:dbl[])
                n248 = global write "rio_Global.vi" "x_l"(w311) -> ()
                n249 = Array Subset(array=w355, index=0, length=w344) -> (w313:dbl[])
                n250 = Array Subset(array=w325, index=0, length=w340) -> (w316:dbl[])
                n251 = Index Array(array=w317, index #1=7 ("index"), index #2=6 ("index"), index #3=9 ("index"), index #4=5 ("index")) -> (element #1=w362:dbl, element #2=w364:dbl, element #3=w366:dbl, element #4=w370:dbl)
                n252 = global write "rio_Global.vi" "x_r"(w313) -> ()
                n253 = global write "rio_Global.vi" "x_c"(w316) -> ()
                n254 = Square(x=w311) -> (x^2=w360:dbl[])
                n255 = Index Array(array=w318, index #1=7 ("index"), index #2=6 ("index"), index #3=9 ("index"), index #4=5 ("index")) -> (element #1=w381:dbl, element #2=w379:dbl, element #3=w377:dbl, element #4=w373:dbl)
                n256 = Index Array(array=w319, index #1=7 ("index"), index #2=6 ("index"), index #3=9 ("index"), index #4=5 ("index")) -> (element #1=w320:dbl, element #2=w334:dbl, element #3=w332:dbl, element #4=w339:dbl)
                n257 = Square(x=w313) -> (x^2=w359:dbl[])
                n258 = Square(x=w316) -> (x^2=w328:dbl[])
                n259 = Compound Arithmetic op=MULTIPLY(w362, w311, w360) -> (w367:dbl[])
                n260 = Compound Arithmetic op=MULTIPLY(w360, w364) -> (w368:dbl[])
                n261 = Compound Arithmetic op=MULTIPLY(w311, w366) -> (w369:dbl[])
                n262 = Compound Arithmetic op=ADD(w367, w368, w369, w370) -> (w312:dbl[])
                n263 = Compound Arithmetic op=MULTIPLY(w381, w313, w359) -> (w376:dbl[])
                n264 = Compound Arithmetic op=MULTIPLY(w359, w379) -> (w375:dbl[])
                n265 = Compound Arithmetic op=MULTIPLY(w313, w377) -> (w374:dbl[])
                n266 = Compound Arithmetic op=MULTIPLY(w320, w316, w328) -> (w331:dbl[])
                n267 = Compound Arithmetic op=MULTIPLY(w328, w334) -> (w330:dbl[])
                n268 = Compound Arithmetic op=MULTIPLY(w316, w332) -> (w329:dbl[])
                n269 = global write "rio_Global.vi" "y_l"(w312) -> ()
                n270 = Compound Arithmetic op=ADD(w376, w375, w374, w373) -> (w314:dbl[])
                n271 = Compound Arithmetic op=ADD(w331, w330, w329, w339) -> (w315:dbl[])
                n272 = global write "rio_Global.vi" "y_r"(w314) -> ()
                n273 = global write "rio_Global.vi" "y_c"(w315) -> ()
              }
              frame #2 {
                n274 = global read "rio_Global.vi" "cmd steer"() -> (w396:dbl)
                n275 = global read "rio_Global.vi" "C_mdps str_ang"() -> (w386:dbl)
                n276 = global read "rio_Global.vi" "C_VS_CAN"() -> (w387:dbl)
                n277 = global read "rio_Global.vi" "ratio"() -> (w395:dbl)
                n278 = global read "rio_Global.vi" "C_VS_CAN"() -> (w385:dbl)
                n279 = global read "rio_Global.vi" "ratio"() -> (w394:dbl)
                n280 = Divide(x=w396, y=w395) -> (x/y=w412:dbl)
                n281 = Multiply(x=w387, y=2.0) -> (x*y=w406:dbl)
                n282 = Divide(x=w386, y=w394) -> (x/y=w425:dbl)
                n283 = Absolute Value(x=w406) -> (abs(x)=w407:dbl)
                n284 = Multiply(x=w385, y=2.0) -> (x*y=w431:dbl)
                n285 = Multiply(x=3.141592653589793, y=w412) -> (x*y=w398:dbl)
                n286 = Absolute Value(x=w431) -> (abs(x)=w430:dbl)
                n287 = Multiply(x=3.141592653589793, y=w425) -> (x*y=w439:dbl)
                n288 = Divide(x=w398, y=180.0) -> (x/y=w400:dbl)
                n289 = Max & Min(x=30.0, y=w407) -> (max(x,y)=w408:dbl)  [unwired: 1 out]
                n290 = global read "rio_Global.vi" "wheel base"() -> (w393:dbl)
                n291 = Tangent(1:w400) -> (0:w410:dbl)
                n292 = Divide(x=w439, y=180.0) -> (x/y=w437:dbl)
                n293 = Max & Min(x=30.0, y=w430) -> (max(x,y)=w429:dbl)  [unwired: 1 out]
                n294 = global read "rio_Global.vi" "wheel base"() -> (w392:dbl)
                n295 = global read "rio_Global.vi" "rear tread width"() -> (w383:dbl)
                n296 = Divide(x=w393, y=w410) -> (x/y=w416:dbl)
                n297 = Round Toward -Infinity(1:w408) -> (0:w403:dbl)
                n298 = Tangent(1:w437) -> (0:w427:dbl)
                n299 = global read "rio_Global.vi" "rear tread width"() -> (w384:dbl)
                n300 = Sign(1:w416) -> (0:w414:dbl)
                n301 = Increment(x=w403) -> (x+1=w405:dbl)
                n302 = Divide(x=w392, y=w427) -> (x/y=w421:dbl)
                n303 = Round Toward -Infinity(1:w429) -> (0:w434:dbl)
                n304 = local read "x_view"() -> (w401:dbl[])
                n305 = Sign(1:w421) -> (0:w423:dbl)
                n306 = Increment(x=w434) -> (x+1=w432:dbl)
                n307 = Compound Arithmetic op=MULTIPLY(w414, w383, 0.5 ("value")) -> (w415:dbl)
                n308 = local read "x_view"() -> (w436:dbl[])
                n309 = Add(x=w416, y=w415) -> (x+y=w418:dbl)
                n310 = Array Subset(array=w401, index=0, length=w405) -> (w411:dbl[])
                n311 = Equal To 0?(x=w410) -> (x = 0?=w417:bool)
                n312 = Compound Arithmetic op=MULTIPLY(w423, w384, 0.5 ("value")) -> (w422:dbl)
                n313 = Add(x=w421, y=w422) -> (x+y=w419:dbl)
                n314 = Equal To 0?(x=w427) -> (x = 0?=w420:bool)
                n315 = case shown="False" w417 {
                  tunnel: w418 -> [w456 _]
                  tunnel: [w446 w461] -> w389
                  tunnel: w411 -> [w444 w463]
                  tunnel: [w442 w463] -> w388
                  frame False {
                    n316 = Square(x=w456) -> (x^2=w460:dbl)
                    n317 = Square(x=w444) -> (x^2=w452:dbl[])
                    n318 = Sign(1:w456) -> (0:w455:dbl)
                    n319 = Absolute Value(x=w456) -> (abs(x)=w458:dbl)
                    n320 = Negate(x=w455) -> (-x=w454:dbl)
                    n321 = Subtract(x=w460, y=w452) -> (x-y=w450:dbl[])
                    n322 = Absolute Value(x=w450) -> (abs(x)=w459:dbl[])
                    n323 = Greater Or Equal To 0?(x=w450) -> (x >= 0?=w449:bool[])
                    n324 = Negate(x=w458) -> (-x=w457:dbl)
                    n325 = Square Root(x=w459) -> (sqrt(x)=w451:dbl[])
                    n326 = Boolean To (0,1)(Boolean=w449) -> (0, 1=w448:i16[])
                    n327 = Add(x=w457, y=w451) -> (x+y=w453:dbl[])
                    n328 = Add Array Elements(numeric array=w448) -> (sum=w443:i16)
                    n329 = Multiply(x=w454, y=w453) -> (x*y=w447:dbl[])
                    n330 = Array Subset(array=w444, index=0, length=w443) -> (w442:dbl[])
                    n331 = Array Subset(array=w447, index=0, length=w443) -> (w446:dbl[])
                  }
                  frame True {
                    n332 = Multiply(x=w463, y=0.0) -> (x*y=w461:dbl[])
                  }
                }
                n333 = Array Subset(array=w436, index=0, length=w432) -> (w426:dbl[])
                n334 = case shown="False" w420 {
                  tunnel: w419 -> [w479 _]
                  tunnel: [w469 w484] -> w390
                  tunnel: w426 -> [w467 w486]
                  tunnel: [w465 w486] -> w391
                  frame False {
                    n335 = Square(x=w479) -> (x^2=w483:dbl)
                    n336 = Square(x=w467) -> (x^2=w475:dbl[])
                    n337 = Sign(1:w479) -> (0:w478:dbl)
                    n338 = Absolute Value(x=w479) -> (abs(x)=w481:dbl)
                    n339 = Negate(x=w478) -> (-x=w477:dbl)
                    n340 = Subtract(x=w483, y=w475) -> (x-y=w473:dbl[])
                    n341 = Absolute Value(x=w473) -> (abs(x)=w482:dbl[])
                    n342 = Greater Or Equal To 0?(x=w473) -> (x >= 0?=w472:bool[])
                    n343 = Negate(x=w481) -> (-x=w480:dbl)
                    n344 = Square Root(x=w482) -> (sqrt(x)=w474:dbl[])
                    n345 = Boolean To (0,1)(Boolean=w472) -> (0, 1=w471:i16[])
                    n346 = Add(x=w480, y=w474) -> (x+y=w476:dbl[])
                    n347 = Add Array Elements(numeric array=w471) -> (sum=w466:i16)
                    n348 = Multiply(x=w477, y=w476) -> (x*y=w470:dbl[])
                    n349 = Array Subset(array=w467, index=0, length=w466) -> (w465:dbl[])
                    n350 = Array Subset(array=w470, index=0, length=w466) -> (w469:dbl[])
                  }
                  frame True {
                    n351 = Multiply(x=w486, y=0.0) -> (x*y=w484:dbl[])
                  }
                }
                n352 = global write "rio_Global.vi" "x_p 2"(w388) -> ()
                n353 = global write "rio_Global.vi" "y_p 2"(w389) -> ()
                n354 = global write "rio_Global.vi" "x_p"(w391) -> ()
                n355 = global write "rio_Global.vi" "y_p"(w390) -> ()
              }
              frame #3 {
                w492 = dynamicdata [] ("Dynamic Data Type")
                n356 = global read "rio_Global.vi" "M_obs"() -> (w488:dbl[][])
                n357 = global read "rio_Global.vi" "M_time"() -> (w487:dbl)
                n358 = Index Array(array=w488, index (col)=17 ("disabled index (col)")) -> (element=w500:dbl[])  [unwired: 1 in]
                n359 = Subtract(x=w500, y=w487) -> (x-y=w499:dbl[])
                n360 = Multiply(x=w499, y=1.0) -> (x*y=w497:dbl[])
                n361 = Absolute Value(x=w497) -> (abs(x)=w496:dbl[])
                n362 = Less?(x=w496, y=1.0) -> (x < y?=w494:bool[])
                n363 = Boolean To (0,1)(Boolean=w494) -> (0, 1=w493:i16[])
                n364 = Add Array Elements(numeric array=w493) -> (sum=w491:i16)
                n365 = for {
                  N: w491 -> [_]
                  tunnel: w488 -> [w536] mode=indexing
                  shift-right: [w518] -> w490
                  shift-left: w492 -> [w520]
                  shift-right: [w516] -> w489
                  shift-left: w492 -> [w515]
                  w506 = 0.0 ("element")
                  w522 = 0.0 ("x0")
                  n366 = Index Array(array=w536, index #1=2 ("index"), index #2=8 ("index"), index #3=9 ("index"), index #4=16 ("index"), index #5=1 ("index")) -> (element #1=w510:dbl, element #2=w505:dbl, element #3=w533:dbl, element #4=w528:dbl, element #5=w511:dbl)
                  n367 = Max & Min(x=w505, y=5.0) -> (min(x,y)=w503:dbl)  [unwired: 1 out]
                  n368 = Multiply(x=w528, y=3.141592653589793) -> (x*y=w526:dbl)
                  n369 = Multiply(x=w533, y=0.5) -> (x*y=w531:dbl)
                  n370 = Negate(x=w531) -> (-x=w530:dbl)
                  n371 = Divide(x=w526, y=180.0) -> (x/y=w521:dbl)
                  n372 = Build Array(w530, w531, w531, w530, w530) -> (w524:dbl[])
                  n373 = Build Array(w506, w506, w503, w503, w506) -> (w523:dbl[])
                  n374 = Negate(x=w510) -> (-x=w509:dbl)
                  n375 = call "rotm_obs_new.vi"("angle[rad]"=w521, "y0"=w522, "x0"=w522, "y"=w523, "x"=w524) -> ("rot*(y-y0) 2"=w514:dbl[], "rot*(x-x0)"=w508:dbl[])  [unwired: 3 in, 2 out]
                  n376 = Add(x=w509, y=w508) -> (x+y=w507:dbl[])
                  n377 = Add(x=w514, y=w511) -> (x+y=w513:dbl[])
                  n378 = call "Convert to Dynamic Data13"("Array"=w507) -> ("Dynamic Data Type"=w519:dynamicdata)  [unwired: 3 in]
                  n379 = call "Convert to Dynamic Data14"("Array"=w513) -> ("Dynamic Data Type"=w517:dynamicdata)  [unwired: 3 in]
                  n380 = Merge Signals(w520, w519) -> (w518:dynamicdata)
                  n381 = Merge Signals(w515, w517) -> (w516:dynamicdata)
                }
              }
              frame #4 {
                n382 = global read "rio_Global.vi" "y_p 2"() -> (w542:dbl[])
                n383 = global read "rio_Global.vi" "y_p"() -> (w543:dbl[])
                n384 = global read "rio_Global.vi" "y_c"() -> (w544:dbl[])
                n385 = global read "rio_Global.vi" "y_r"() -> (w546:dbl[])
                n386 = global read "rio_Global.vi" "y_l"() -> (w545:dbl[])
                n387 = global read "rio_Global.vi" "x_p 2"() -> (w537:dbl[])
                n388 = global read "rio_Global.vi" "x_p"() -> (w538:dbl[])
                n389 = global read "rio_Global.vi" "x_c"() -> (w539:dbl[])
                n390 = global read "rio_Global.vi" "x_r"() -> (w541:dbl[])
                n391 = call "Convert to Dynamic Data"("Array"=w546) -> ("Dynamic Data Type"=w567:dynamicdata)  [unwired: 3 in]
                n392 = call "Convert to Dynamic Data3"("Array"=w545) -> ("Dynamic Data Type"=w564:dynamicdata)  [unwired: 3 in]
                n393 = call "Convert to Dynamic Data5"("Array"=dbl[] [-0.94, 0.94, 0.94, -0.94, -0.94] ("appended array 2")) -> ("Dynamic Data Type"=w559:dynamicdata)  [unwired: 3 in]
                n394 = call "Convert to Dynamic Data7"("Array"=w544) -> ("Dynamic Data Type"=w554:dynamicdata)  [unwired: 3 in]
                n395 = call "Convert to Dynamic Data10"("Array"=w543) -> ("Dynamic Data Type"=w551:dynamicdata)  [unwired: 3 in]
                n396 = call "Convert to Dynamic Data12"("Array"=w542) -> ("Dynamic Data Type"=w547:dynamicdata)  [unwired: 3 in]
                n397 = Add(x=dbl[] [-3.5, -3.5, 1.2, 1.2, -3.5] ("appended array"), y=0.3) -> (x+y=w556:dbl[])
                n398 = global read "rio_Global.vi" "x_l"() -> (w540:dbl[])
                n399 = Merge Signals(w567, w564, w559, w554, w551, w547, w548) -> (w561:dynamicdata)
                n400 = call "Convert to Dynamic Data2"("Array"=w541) -> ("Dynamic Data Type"=w566:dynamicdata)  [unwired: 3 in]
                n401 = call "Convert to Dynamic Data6"("Array"=w556) -> ("Dynamic Data Type"=w558:dynamicdata)  [unwired: 3 in]
                n402 = call "Convert to Dynamic Data8"("Array"=w539) -> ("Dynamic Data Type"=w553:dynamicdata)  [unwired: 3 in]
                n403 = call "Convert to Dynamic Data9"("Array"=w538) -> ("Dynamic Data Type"=w552:dynamicdata)  [unwired: 3 in]
                n404 = call "Convert to Dynamic Data11"("Array"=w537) -> ("Dynamic Data Type"=w549:dynamicdata)  [unwired: 3 in]
                n405 = call "Convert to Dynamic Data4"("Array"=w540) -> ("Dynamic Data Type"=w562:dynamicdata)  [unwired: 3 in]
                n406 = Merge Signals(w566, w562, w558, w553, w552, w549, w550) -> (w563:dynamicdata)
                n407 = call "Build XY Graph"("Y Input"=w563, "X Input"=w561) -> ("XY Graph"=→"XY Graph":cluster{"X":dbl[], "Y":dbl[]}[])  [unwired: 8 in, 1 out]
              }
            }
          }
        }
      }
    }
  }
  n408 = flat-sequence {
    tunnel: [dbl[] [0.0, 0.0, 0.0, 0.0, 0.0] ("pos(i)")] -> w1
    tunnel: w1 -> [w584]
    frame #0 {
      w575 = FALSE ("get heading")
      w576 = u64 1
      w573 = 0.0 ("dh_hat")
      w579 = 4 ("map")
      n409 = local write "GPS init"(w575) -> ()
      n410 = call "getecefdcmref.vi"("map"=w579) -> ("XYZ"=→"ecef ref":dbl[])  [unwired: 10 in, 4 out]
      n411 = while {
        shift-right: [w582] -> w571
        shift-left: refnum<visa-resource-name> "USB0::0x1546::0x01A8::NI-VISA-1003::1::RAW" ("VISA resource name") -> [w583]
        stop <- w581 continue-if-true
        n412 = VISA Open(VISA resource name=w583) -> (VISA resource name=w582:refnum<visa-resource-name>, error out=w581:errorcluster)  [unwired: 4 in]
      }
      n413 = VISA Clear(VISA resource name=w571) -> (VISA resource name out=w569:refnum<visa-resource-name>)  [unwired: 1 in, 1 out]
      n414 = property class="Instr"(reference=w569, "General Settings:Timeout Value"=u32 10) -> (reference out=→"gps1":refnum<visa-resource-name>)  [unwired: 1 in, 1 out]
      "map" <- w579
      "vgain" <- 1.0 ("initH")
      "vcount" <- w576
      "hbias" <- w573
      "hcount" <- w576
      "get heading" <- w575
      "get position" <- w575
      "heading error" <- w573
      "h_gps" <- w573
      "rt" <- w573
      "pos error" <- w573
      "POS init" <- TRUE ("POS init")
    }
    frame #1 {
      (unwired) FALSE
      n415 = while {
        stop <- FALSE stop-if-true
        n416 = flat-sequence {
          tunnel: [w587] -> w585
          tunnel: w585 -> [w654]
          frame #0 {
            n417 = local read "gps1"() -> (w590:refnum<visa-resource-name>)
            n418 = VISA Read(VISA resource name=w590, byte count=u32 100) -> (read buffer=w588:string, return count=w587:u32)  [unwired: 1 in, 2 out]
            n419 = case shown="\"True\", Default" w588 {
              selector: w588 -> [_ w591]
              frame "" {
              }
              frame "True", Default {
                n420 = local read "ecef ref"() -> (w592:dbl[])
                n421 = call "nmea.vi"("ecef ref"=w592, "NMEA"=w591) -> ("output"=w594:dbl[], "type"=w593:u32)  [unwired: 8 in]
                n422 = case shown="1" w593 {
                  tunnel: w594 -> [_ w596 w629]
                  frame 0, Default {
                  }
                  frame 1 {
                    n423 = global write "rio_Global.vi" "gps_pos 1"(w596) -> ()
                    n424 = Index Array(array=w596, index=1) -> (element=w598:dbl)
                    n425 = Not Equal To 0?(x=w598) -> (x != 0?=w595:bool)
                    n426 = case shown="True" w595 {
                      tunnel: w596 -> [_ w618]
                      frame False {
                      }
                      frame True {
                        n427 = Get Date/Time In Seconds() -> (seconds since 1Jan1904=w603:timestamp)
                        n428 = To Double Precision Float(number=w603) -> (double precision float=w602:dbl)
                        n429 = global read "rio_Global.vi" "LCM_GGA_T"() -> (w627:T7)
                        n430 = Array To Cluster(array=w618) -> (cluster=w626:T8)
                        n431 = Unbundle By Name(w627) -> ("hash"=w623:i64)
                        n432 = Multiply(x=w602, y=1000000.0) -> (x*y=w600:dbl)
                        n433 = Unbundle(w626) -> ("output[0]"=w628:dbl, "output[2]"=w617:dbl, "output[3]"=w616:dbl, "output[4]"=w615:dbl, "output[6]"=w614:dbl, "output[7]"=w612:dbl, "output[8]"=w610:dbl, "output[9]"=w608:dbl, "output[12]"=w607:dbl, "output[13]"=w606:dbl, "output[14]"=w605:dbl)  [unwired: 4 out]
                        n434 = call "hash.vi"("input"=w623) -> ("output"=w622:i64)  [unwired: 10 in]
                        n435 = To Quad Integer(1:w600) -> (0:w599:i64)
                        n436 = To Long Integer(number=w614) -> (32bit integer=w613:i32)
                        n437 = To Long Integer(number=w612) -> (32bit integer=w611:i32)
                        n438 = To Long Integer(number=w610) -> (32bit integer=w609:i32)
                        n439 = local read "map"() -> (w604:i32)
                        n440 = Bundle(cluster=w627, "hash"=w622, "sys time"=w599, "time"=w628, "x"=w617, "y"=w616, "h"=w615, "numSV"=w613, "postype"=w611, "lag"=w609, "hordev"=w608, "lat"=w607, "lon"=w606, "hgt"=w605, "map_idx"=w604) -> (w624:T7)
                        n441 = Flatten To String(anything=w624, prepend array or string size? (T)=FALSE) -> (data string=w620:string)  [unwired: 2 in, 2 out]
                        n442 = global read "rio_Global.vi" "LCM"() -> (w619:T2)
                        n443 = call "LCM_send.vi"("DATA"=w620, "ID"="GGA_1", "LCM"=w619) -> ()  [unwired: 6 in, 3 out]
                      }
                    }
                  }
                  frame 2 {
                    n444 = global write "rio_Global.vi" "gps_vel 1"(w629) -> ()
                    n445 = flat-sequence {
                      tunnel: w629 -> [w631]
                      frame #0 {
                        n446 = Index Array(array=w631, index=1) -> (element=w633:dbl)
                        n447 = Not Equal To 0?(x=w633) -> (x != 0?=w630:bool)
                        n448 = case shown="True" w630 {
                          tunnel: w631 -> [_ w652]
                          frame False {
                          }
                          frame True {
                            n449 = Get Date/Time In Seconds() -> (seconds since 1Jan1904=w638:timestamp)
                            n450 = To Double Precision Float(number=w638) -> (double precision float=w637:dbl)
                            n451 = global read "rio_Global.vi" "LCM_RMC_T"() -> (w653:T9)
                            n452 = Unbundle By Name(w653) -> ("hash"=w649:i64)
                            n453 = Multiply(x=w637, y=1000000.0) -> (x*y=w635:dbl)
                            n454 = Array To Cluster(array=w652) -> (cluster=w651:T10)
                            n455 = call "hash.vi"("input"=w649) -> ("output"=w648:i64)  [unwired: 10 in]
                            n456 = To Quad Integer(1:w635) -> (0:w634:i64)
                            n457 = Unbundle(w651) -> ("output[0]"=w643:dbl, "output[2]"=w642:dbl, "output[4]"=w641:dbl, "output[5]"=w640:dbl, "output[6]"=w639:dbl)  [unwired: 2 out]
                            n458 = Bundle(cluster=w653, "hash"=w648, "sys time"=w634, "time"=w643, "speed"=w642, "heading"=w641, "lat"=w640, "lon"=w639) -> (w644:T9)
                            n459 = Flatten To String(anything=w644, prepend array or string size? (T)=FALSE) -> (data string=w646:string)  [unwired: 2 in, 2 out]
                            n460 = global read "rio_Global.vi" "LCM"() -> (w645:T2)
                            n461 = call "LCM_send.vi"("DATA"=w646, "ID"="RMC_1", "LCM"=w645) -> ()  [unwired: 6 in, 3 out]
                          }
                        }
                      }
                    }
                  }
                }
              }
            }
          }
          frame #1 {
            n462 = case shown="Default" w654 {
              frame Default {
                n463 = Wait (ms)(milliseconds to wait=u32 20) -> ()  [unwired: 1 out]
              }
              frame 0 {
              }
            }
          }
        }
      }
      n464 = while {
        shift-right: [w656] -> _
        shift-left: w584 -> [w657]
        stop <- FALSE stop-if-true
        n465 = flat-sequence {
          tunnel: [w668] -> w660
          tunnel: w657 -> [w668]
          tunnel: w660 -> [w671]
          tunnel: [w670] -> w659
          tunnel: [w670] -> w658
          tunnel: [w1084] -> w656
          tunnel: w659 -> [w1085]
          tunnel: w658 -> [w1084]
          frame #0 {
            n466 = global read "rio_Global.vi" "C_ts"() -> (→"dt":dbl)
            n467 = Wait Until Next ms Multiple(millisecond multiple=u32 10) -> (millisecond timer value=w666:u32)
            n468 = feedback #6(w666) -> (w665:u32)
            n469 = feedback-in #6(w666) -> ()
            n470 = Subtract(x=w666, y=w665) -> (x-y=w664:u32)
            n471 = To Long Integer(number=w664) -> (32bit integer=→"Pos_time 10":i32)
          }
          frame #1 {
            n472 = flat-sequence {
              tunnel: w671 -> [w678]
              tunnel: [w678] -> w669
              tunnel: [w801] -> w670
              tunnel: w669 -> [w802]
              frame #0 {
                n473 = disable-structure shown="Enabled" {
                  disable-tunnel: [w698 w699] -> w673
                  disable-tunnel: [w679 w700] -> w672
                  frame Disabled {
                    n474 = global read "rio_Global.vi" "gps_pos 1"() -> (w695:dbl[])
                    n475 = global read "rio_Global.vi" "gps_pos 2"() -> (w682:dbl[])
                    n476 = Add(x=w695, y=w682) -> (x+y=w697:dbl[])
                    n477 = Index Array(array=w695, index #1=0 ("index")) -> (element #1=w694:dbl, element #2=w693:dbl)  [unwired: 1 in]
                    n478 = Index Array(array=w682, index #1=0 ("index")) -> (element #1=w683:dbl, element #2=w684:dbl)  [unwired: 1 in]
                    n479 = feedback #7(w694) -> (w692:dbl)
                    n480 = feedback-in #7(w694) -> ()
                    n481 = feedback #8(w683) -> (w685:dbl)
                    n482 = feedback-in #8(w683) -> ()
                    n483 = Not Equal?(x=w694, y=w692) -> (x != y?=w691:bool)
                    n484 = Not Equal?(x=w683, y=w685) -> (x != y?=w686:bool)
                    n485 = Not Equal To 0?(x=w693) -> (x != 0?=w690:bool)
                    n486 = Not Equal To 0?(x=w684) -> (x != 0?=w687:bool)
                    n487 = And(x=w691, y=w690) -> (x .and. y?=w680:bool)
                    n488 = And(x=w686, y=w687) -> (x .and. y?=w681:bool)
                    n489 = And(x=w680, y=w681) -> (x .and. y?=w698:bool)
                    n490 = Multiply(x=w697, y=0.5) -> (x*y=w679:dbl[])
                  }
                  frame Enabled {
                    n491 = global read "rio_Global.vi" "gps_pos 1"() -> (w700:dbl[])
                    n492 = Index Array(array=w700, index #1=0 ("index")) -> (element #1=w706:dbl, element #2=w705:dbl)  [unwired: 1 in]
                    n493 = feedback #9(w706) -> (w704:dbl)
                    n494 = feedback-in #9(w706) -> ()
                    n495 = Not Equal?(x=w706, y=w704) -> (x != y?=w703:bool)
                    n496 = Not Equal To 0?(x=w705) -> (x != 0?=w702:bool)
                    n497 = And(x=w703, y=w702) -> (x .and. y?=w699:bool)
                  }
                }
                "pos_gps" <- w672
                n498 = disable-structure shown="Enabled" {
                  disable-tunnel: [w752 w783] -> w677
                  disable-tunnel: [w751 w762] -> w676
                  disable-tunnel: [w723 w773] -> w675
                  disable-tunnel: [w711 w768] -> w674
                  frame Disabled {
                    n499 = global read "rio_Global.vi" "gps_vel 1"() -> (w750:dbl[])
                    n500 = global read "rio_Global.vi" "gps_vel 2"() -> (w729:dbl[])
                    n501 = Index Array(array=w750, index #1=0 ("index"), index #2=1 ("index"), index #3=4 ("index"), index #4=2 ("index")) -> (element #1=w741:dbl, element #2=w746:dbl, element #3=w743:dbl, element #4=w715:dbl)
                    n502 = Index Array(array=w729, index #1=0 ("index"), index #2=1 ("index"), index #3=4 ("index"), index #4=2 ("index")) -> (element #1=w738:dbl, element #2=w733:dbl, element #3=w736:dbl, element #4=w714:dbl)
                    n503 = global read "rio_Global.vi" "C_VS_CAN"() -> (w708:dbl)
                    n504 = global read "rio_Global.vi" "C_VS_CAN"() -> (w755:dbl)
                    n505 = Add(x=w715, y=w714) -> (x+y=w713:dbl)
                    n506 = Not Equal To 0?(x=w733) -> (x != 0?=w734:bool)
                    n507 = call "angleconv.vi"("deg"=w743) -> ("rad"=w726:dbl)  [unwired: 9 in, 1 out]
                    n508 = call "angleconv.vi"("deg"=w736) -> ("rad"=w725:dbl)  [unwired: 9 in, 1 out]
                    n509 = feedback #10(0.0 ("Real Matrix Element")) -> (w740:dbl)
                    n510 = feedback-in #10(w741) -> ()
                    n511 = feedback #11(0.0 ("Real Matrix Element")) -> (w739:dbl)
                    n512 = feedback-in #11(w738) -> ()
                    n513 = Not Equal?(x=w741, y=w740) -> (x != y?=w747:bool)
                    n514 = Not Equal?(x=w738, y=w739) -> (x != y?=w732:bool)
                    n515 = Not Equal To 0?(x=w746) -> (x != 0?=w745:bool)
                    n516 = Greater Or Equal To 0?(x=w755) -> (x >= 0?=w756:bool)
                    n517 = Absolute Value(x=w708) -> (abs(x)=w707:dbl)
                    n518 = Multiply(x=w713, y=0.5) -> (x*y=w722:dbl)
                    n519 = call "headingweightsum.vi"("a"=0.5, "h1"=w725, "h2"=w726) -> ("a*h2+(1-a)*h1"=w754:dbl)  [unwired: 8 in]
                    n520 = And(x=w747, y=w745) -> (x .and. y?=w728:bool)
                    n521 = And(x=w732, y=w734) -> (x .and. y?=w727:bool)
                    n522 = Divide(x=w722, y=w707) -> (x/y=w723:dbl)
                    n523 = Select(t=0.0, s=w756, f=3.141592653589793) -> (s? t:f=w753:dbl)
                    n524 = Decrement(x=w723) -> (x-1=w719:dbl)
                    n525 = call "headingoperater.vi"("h1"=w753, "h2"=w754) -> ("h2-h1"=w752:dbl)  [unwired: 8 in, 1 out]
                    n526 = And(x=w728, y=w727) -> (x .and. y?=w751:bool)
                    n527 = Absolute Value(x=w719) -> (abs(x)=w720:dbl)
                    n528 = Greater?(x=w707, y=15.0) -> (0:w709:bool)
                    n529 = Less?(x=w720, y=0.05) -> (x < y?=w712:bool)
                    n530 = Compound Arithmetic op=AND(w709, w712, w751) -> (w711:bool)
                  }
                  frame Enabled {
                    n531 = global read "rio_Global.vi" "gps_vel 1"() -> (w782:dbl[])
                    n532 = global read "rio_Global.vi" "C_VS_CAN"() -> (w766:dbl)
                    n533 = global read "rio_Global.vi" "C_VS_CAN"() -> (w785:dbl)
                    n534 = Index Array(array=w782, index #1=0 ("index"), index #2=1 ("index"), index #3=4 ("index"), index #4=2 ("index")) -> (element #1=w761:dbl, element #2=w778:dbl, element #3=w775:dbl, element #4=w764:dbl)
                    n535 = Greater Or Equal To 0?(x=w785) -> (x >= 0?=w786:bool)
                    n536 = Absolute Value(x=w766) -> (abs(x)=w765:dbl)
                    n537 = feedback #12(w761) -> (w774:dbl)
                    n538 = feedback-in #12(w761) -> ()
                    n539 = Divide(x=w764, y=w765) -> (x/y=w773:dbl)
                    n540 = call "angleconv.vi"("deg"=w775) -> ("rad"=w763:dbl)  [unwired: 9 in, 1 out]
                    n541 = Select(t=0.0, s=w786, f=3.141592653589793) -> (s? t:f=w784:dbl)
                    n542 = Not Equal?(x=w761, y=w774) -> (x != y?=w779:bool)
                    n543 = Not Equal To 0?(x=w778) -> (x != 0?=w777:bool)
                    n544 = Decrement(x=w773) -> (x-1=w770:dbl)
                    n545 = call "headingoperater.vi"("h1"=w784, "h2"=w763) -> ("h2-h1"=w783:dbl)  [unwired: 8 in, 1 out]
                    n546 = And(x=w779, y=w777) -> (x .and. y?=w762:bool)
                    n547 = Absolute Value(x=w770) -> (abs(x)=w771:dbl)
                    n548 = Greater?(x=w765, y=15.0) -> (0:w759:bool)
                    n549 = Less?(x=w771, y=0.05) -> (x < y?=w760:bool)
                    n550 = Compound Arithmetic op=AND(w762, w760, w759) -> (w768:bool)
                  }
                }
                n551 = local write "get position"(w673) -> ()
                n552 = local write "h_gps"(w677) -> ()
                n553 = local write "get heading"(w676) -> ()
                n554 = case shown="True" w674 {
                  tunnel: w675 -> [_ w796]
                  frame False {
                  }
                  frame True {
                    w790 = u64 18446744073709551615
                    n555 = local read "vcount"() -> (w793:u64)
                    n556 = local read "vgain"() -> (w798:dbl)
                    n557 = Increment(x=w793) -> (x+1=w792:u64)
                    n558 = Not Equal?(x=w793, y=w790) -> (x != y?=w791:bool)
                    n559 = Multiply(x=w798, y=w793) -> (x*y=w797:dbl)
                    n560 = Add(x=w796, y=w797) -> (x+y=w795:dbl)
                    n561 = Select(t=w792, s=w791, f=w790) -> (s? t:f=w789:u64)
                    n562 = Divide(x=w795, y=w789) -> (x/y=w794:dbl)
                    n563 = local write "vcount"(w789) -> ()
                    n564 = local write "vgain"(w794) -> ()
                  }
                }
              }
              frame #1 {
                n565 = local read "dt"() -> (w800:dbl)
                n566 = Greater Than 0?(x=w800) -> (x > 0?=w799:bool)
                n567 = case shown="True" w799 {
                  tunnel: w802 -> [w803 w806]
                  tunnel: [w803 w805] -> w801
                  frame False {
                  }
                  frame True {
                    n568 = flat-sequence {
                      tunnel: w806 -> [w840]
                      tunnel: [w818] -> w804
                      tunnel: [w868] -> w805
                      tunnel: w804 -> [w867]
                      frame #0 {
                        n569 = global read "rio_Global.vi" "C_VS_CAN"() -> (w808:dbl)
                        n570 = Equal To 0?(x=w808) -> (x = 0?=w810:bool)
                        n571 = case shown="True" w810 {
                          tunnel: [w842 _] -> w809
                          frame False {
                            n572 = global read "rio_Global.vi" "C_yaw_rate"() -> (w841:dbl)
                            n573 = local read "hbias"() -> (w845:dbl)
                            n574 = Subtract(x=w841, y=w845) -> (x-y=w843:dbl)
                            n575 = Negate(x=w843) -> (-x=w844:dbl)
                            n576 = call "angleconv.vi"("deg"=w844) -> ("rad"=w842:dbl)  [unwired: 9 in, 1 out]
                          }
                          frame True {
                            w849 = u64 18446744073709551615
                            n577 = local read "hcount"() -> (w852:u64)
                            n578 = local read "hbias"() -> (w855:dbl)
                            n579 = Increment(x=w852) -> (x+1=w851:u64)
                            n580 = global read "rio_Global.vi" "C_yaw_rate"() -> (w846:dbl)
                            n581 = Not Equal?(x=w852, y=w849) -> (x != y?=w850:bool)
                            n582 = Multiply(x=w855, y=w852) -> (x*y=w854:dbl)
                            n583 = Add(x=w846, y=w854) -> (x+y=w853:dbl)
                            n584 = Select(t=w851, s=w850, f=w849) -> (s? t:f=w848:u64)
                            n585 = local write "hcount"(w848) -> ()
                            n586 = Divide(x=w853, y=w848) -> (x/y=w847:dbl)
                            n587 = local write "hbias"(w847) -> ()
                          }
                        }
                        n588 = global read "rio_Global.vi" "C_VS_CAN"() -> (w807:dbl)
                        n589 = local read "vgain"() -> (w813:dbl)
                        n590 = Multiply(x=w807, y=w813) -> (x*y=w812:dbl)
                        n591 = Divide(x=w812, y=3.6) -> (x/y=w811:dbl)
                        n592 = Index Array(array=w840, index #1=0 ("index"), index #2=3 ("index"), index #3=1 ("index"), index #4=3 ("index")) -> (element #1=w834:dbl, element #2=w832:dbl, element #3=w828:dbl, element #4=w823:dbl)
                        n593 = local read "dt"() -> (w837:dbl)
                        n594 = local read "dt"() -> (w821:dbl)
                        n595 = Multiply(x=w811, y=w837) -> (x*y=w833:dbl)
                        n596 = Multiply(x=w821, y=w809) -> (x*y=w814:dbl)
                        n597 = Cosine(x=w832) -> (cos(x)=w838:dbl)
                        n598 = Sine(x=w832) -> (sin(x)=w831:dbl)
                        n599 = Multiply(x=w838, y=w833) -> (x*y=w835:dbl)
                        n600 = Multiply(x=w833, y=w831) -> (x*y=w830:dbl)
                        n601 = local write "rt"(w814) -> ()
                        n602 = Add(x=w834, y=w835) -> (x+y=w827:dbl)
                        n603 = Add(x=w830, y=w828) -> (x+y=w826:dbl)
                        n604 = call "headingoperater.vi"("h1"=w814, "h2"=w823) -> ("h2+h1"=w822:dbl)  [unwired: 8 in, 1 out]
                        n605 = Build Array(w827, w826, w811, w822, w809) -> (w818:dbl[])
                        n606 = Index Array(array=w818, index=3) -> (element=w817:dbl)
                        n607 = local read "h_gps"() -> (w816:dbl)
                        n608 = call "headingoperater.vi"("h1"=w817, "h2"=w816) -> ("h2-h1"=w820:dbl)  [unwired: 8 in, 1 out]
                        n609 = Absolute Value(x=w820) -> (abs(x)=w815:dbl)
                        n610 = local write "heading error"(w815) -> ()
                      }
                      frame #1 {
                        n611 = local read "get heading"() -> (w875:bool)
                        n612 = local read "get position"() -> (w874:bool)
                        n613 = local read "POS init"() -> (w860:bool)
                        n614 = case shown="False" w860 {
                          tunnel: w875 -> [w878 w885]
                          tunnel: w874 -> [w882 w884]
                          tunnel: [w876 w883] -> w870
                          frame False {
                            n615 = local read "heading error"() -> (w879:dbl)
                            n616 = Less?(x=w879, y=0.05) -> (x < y?=w880:bool)
                            n617 = And(x=w878, y=w880) -> (x .and. y?=w877:bool)
                            n618 = Or(x=w877, y=w882) -> (x .or. y?=w876:bool)
                          }
                          frame True {
                            n619 = disable-structure shown="Enabled" {
                              disable-tunnel: w885 -> [w888 w890]
                              disable-tunnel: w884 -> [w887 w889]
                              disable-tunnel: [w886 w891] -> w883
                              frame Disabled {
                                n620 = And(x=w888, y=w887) -> (x .and. y?=w886:bool)
                              }
                              frame Enabled {
                                n621 = Or(x=w890, y=w889) -> (x .or. y?=w891:bool)
                              }
                            }
                          }
                        }
                        n622 = global read "rio_Global.vi" "C_VS_CAN"() -> (w873:dbl)
                        n623 = local read "heading error"() -> (w863:dbl)
                        n624 = Absolute Value(x=w873) -> (abs(x)=w872:dbl)
                        n625 = local read "POS init"() -> (w861:bool)
                        n626 = Greater?(x=w872, y=5.0) -> (0:w869:bool)
                        n627 = Less?(x=w863, y=1.0) -> (x < y?=w862:bool)
                        n628 = Or(x=w862, y=w861) -> (x .or. y?=w864:bool)
                        n629 = And(x=w870, y=w869) -> (x .and. y?=w865:bool)
                        n630 = And(x=w865, y=w864) -> (x .and. y?=w858:bool)
                        n631 = Select(t=FALSE, s="GPS init", f=w858) -> (s? t:f=w857:bool)
                        n632 = case shown="True" w857 {
                          tunnel: [w895 w924] -> w868
                          tunnel: w867 -> [w896 w927]
                          frame False {
                            n633 = global read "rio_Global.vi" "C_VS_CAN"() -> (w899:dbl)
                            n634 = local read "POS init"() -> (w898:bool)
                            n635 = Equal To 0?(x=w899) -> (x = 0?=w897:bool)
                            n636 = local read "GPS init"() -> (w892:bool)
                            n637 = And(x=w898, y=w897) -> (x .and. y?=w894:bool)
                            n638 = Or(x=w894, y=w892) -> (x .or. y?=w893:bool)
                            n639 = case shown="True" w893 {
                              tunnel: w896 -> [w900 w901]
                              tunnel: [w900 w903] -> w895
                              tunnel: w892 -> [_ w902]
                              frame False {
                              }
                              frame True {
                                n640 = case shown="False" w902 {
                                tunnel: [w914 w923] -> w903
                                tunnel: w901 -> [w909 w917]
                                frame True {
                                n641 = Index Array(array=w909, index #1=2 ("index")) -> (element #2=w904:dbl, element #3=w907:dbl)  [unwired: 2 in, 1 out]
                                n642 = local read "pos_gps"() -> (w910:dbl[])
                                n643 = local write "GPS init"(FALSE ("GPS init")) -> ()
                                n644 = Index Array(array=w910, index #1=2 ("index")) -> (element #1=w912:dbl, element #2=w911:dbl)  [unwired: 1 in]
                                n645 = local read "h_gps"() -> (w905:dbl)
                                n646 = Build Array(w912, w911, w904, w905, w907) -> (w914:dbl[])
                                }
                                frame False {
                                w916 = 0.0 ("element")
                                n647 = Index Array(array=w917, index=3) -> (element=w915:dbl)
                                n648 = local read "pos_gps"() -> (w919:dbl[])
                                n649 = Index Array(array=w919, index #1=2 ("index")) -> (element #1=w921:dbl, element #2=w920:dbl)  [unwired: 1 in]
                                n650 = Build Array(w921, w920, w916, w915, w916) -> (w923:dbl[])
                                }
                                }
                              }
                            }
                          }
                          frame True {
                            n651 = flat-sequence {
                              tunnel: w927 -> [w928]
                              tunnel: [w928] -> w926
                              tunnel: w926 -> [w969]
                              tunnel: [w969] -> w925
                              tunnel: w925 -> [w996]
                              tunnel: [w1000] -> w924
                              frame #0 {
                                w937 = 0.0 ("element")
                                w941 = 0.0 ("element")
                                w943 = 0.0 ("element")
                                w945 = 0.0 ("element")
                                w947 = 0.0 ("element")
                                n652 = Index Array(array=w928, index #1=3 ("index"), index #2=2 ("index"), index #3=3 ("index"), index #4=2 ("index")) -> (element #1=w957:dbl, element #2=w959:dbl, element #3=w962:dbl, element #4=w951:dbl)
                                n653 = Negate(x=w959) -> (-x=w958:dbl)
                                n654 = Sine & Cosine(0:w962) -> (1:w954:dbl, 2:w952:dbl)
                                n655 = Multiply(x=w958, y=w954) -> (x*y=w955:dbl)
                                n656 = Multiply(x=w952, y=w951) -> (x*y=w950:dbl)
                                n657 = Cosine(x=w957) -> (cos(x)=w956:dbl)
                                n658 = Build Array(w947, w947, w956, w955, 0.0 ("element")) -> (w949:dbl[])
                                n659 = Build Array(w945, w945, w954, w950, 0.0 ("element")) -> (w948:dbl[])
                                n660 = Build Array(w943, w943, w943, w943, w943) -> (w942:dbl[])
                                n661 = Build Array(w941, w941, w941, w941, 1.0 ("element")) -> (w939:dbl[])
                                n662 = Build Array(w937, w937, w937, w937, w937) -> (w938:dbl[])
                                n663 = Build Array(w949, w948, w942, w939, w938) -> (w935:dbl[][])
                                n664 = call-poly <vilib>:"Array To Matrix.vi"("Real 2D Array"=w935) -> ("Real Matrix"=w933:T11)
                                n665 = global read "rio_Global.vi" "P"() -> (w936:T11)
                                n666 = Transpose Matrix(1:w933) -> (0:w932:T11)
                                n667 = call-poly <vilib>:"Multiply.vi"("Real Matrix B"=w936, "Real Matrix A"=w933) -> ("A * B"=w934:T11)
                                n668 = call-poly <vilib>:"Multiply.vi"("Real Matrix B"=w932, "Real Matrix A"=w934) -> ("A * B"=w931:T11)
                                n669 = global read "rio_Global.vi" "Q"() -> (w930:T11)
                                n670 = call-poly <vilib>:"Add.vi"("Real Matrix B"=w930, "Real Matrix A"=w931) -> ("A + B"=w929:T11)
                                n671 = global write "rio_Global.vi" "Pp"(w929) -> ()
                              }
                              frame #1 {
                                n672 = global read "rio_Global.vi" "Pp"() -> (w994:T11)
                                n673 = global read "rio_Global.vi" "H"() -> (w993:T11)
                                n674 = Array Subset(array=w969, index=0, length=2) -> (w976:dbl[])
                                n675 = local read "pos_gps"() -> (w972:dbl[])
                                n676 = call-poly <vilib>:"Multiply.vi"("Real Matrix B"=w994, "Real Matrix A"=w993) -> ("A * B"=w992:T11)
                                n677 = Transpose Matrix(1:w993) -> (0:w991:T11)
                                n678 = call-poly <vilib>:"Multiply.vi"("Real Matrix B"=w991, "Real Matrix A"=w992) -> ("A * B"=w990:T11)
                                n679 = Array Subset(array=w972, index=2, length=2) -> (w975:dbl[])
                                n680 = Subtract(x=w975, y=w976) -> (x-y=w977:dbl[])
                                n681 = global read "rio_Global.vi" "H"() -> (w988:T11)
                                n682 = global read "rio_Global.vi" "R"() -> (w989:T11)
                                n683 = global read "rio_Global.vi" "Pp"() -> (w987:T11)
                                n684 = call-poly <vilib>:"Add.vi"("Real Matrix B"=w989, "Real Matrix A"=w990) -> ("A + B"=w984:T11)
                                n685 = Square(x=w977) -> (x^2=w978:dbl[])
                                n686 = Transpose Matrix(1:w988) -> (0:w986:T11)
                                n687 = local read "heading error"() -> (w981:dbl)
                                n688 = call-poly <vilib>:"Multiply.vi"("Real Matrix B"=w986, "Real Matrix A"=w987) -> ("A * B"=w985:T11)
                                n689 = Add Array Elements(numeric array=w978) -> (sum=w979:dbl)
                                n690 = call-poly <vilib>:"Inverse Matrix.vi"("Input Matrix"=w984) -> ("Inverse Matrix"=w983:T11)  [unwired: 1 in, 1 out]
                                n691 = call-poly <vilib>:"Multiply.vi"("Real Matrix B"=w983, "Real Matrix A"=w985) -> ("A * B"=w982:T11)
                                n692 = Square Root(x=w979) -> (sqrt(x)=w968:dbl)
                                n693 = global write "rio_Global.vi" "K"(w982) -> ()
                                n694 = Less?(x=w968, y=2.5) -> (x < y?=w965:bool)
                                n695 = Less?(x=w981, y=0.05) -> (x < y?=w966:bool)
                                n696 = And(x=w966, y=w965) -> (x .and. y?=w964:bool)
                                n697 = case shown="True" w964 {
                                frame False {
                                }
                                frame True {
                                n698 = local write "POS init"(FALSE ("Kalman init")) -> ()
                                }
                                }
                              }
                              frame #2 {
                                n699 = disable-structure shown="Enabled" {
                                disable-tunnel: [w1012 w1013] -> w999
                                frame Disabled {
                                n700 = local read "get heading"() -> (w1012:bool)
                                }
                                frame Enabled {
                                n701 = local read "heading error"() -> (w1016:dbl)
                                n702 = local read "POS init"() -> (w1014:bool)
                                n703 = Less?(x=w1016, y=0.1) -> (x < y?=w1015:bool)
                                n704 = Or(x=w1015, y=w1014) -> (x .or. y?=w1013:bool)
                                }
                                }
                                n705 = disable-structure shown="Enabled" {
                                disable-tunnel: [w1018 w1020] -> w998
                                disable-tunnel: w996 -> [_ w1029]
                                frame Disabled {
                                n706 = local read "get position"() -> (w1018:bool)
                                }
                                frame Enabled {
                                n707 = Array Subset(array=w1029, index=0, length=2) -> (w1027:dbl[])
                                n708 = local read "pos_gps"() -> (w1032:dbl[])
                                n709 = Array Subset(array=w1032, index=2, length=2) -> (w1028:dbl[])
                                n710 = disable-structure shown="Enabled" {
                                disable-tunnel: [w1035 TRUE ("Kalman init")] -> w1022
                                frame Disabled {
                                n711 = local read "POS init"() -> (w1035:bool)
                                }
                                frame Enabled {
                                }
                                }
                                n712 = Subtract(x=w1028, y=w1027) -> (x-y=w1026:dbl[])
                                n713 = Square(x=w1026) -> (x^2=w1025:dbl[])
                                n714 = Add Array Elements(numeric array=w1025) -> (sum=w1024:dbl)
                                n715 = Square Root(x=w1024) -> (sqrt(x)=w1019:dbl)
                                n716 = local write "pos error"(w1019) -> ()
                                n717 = Less?(x=w1019, y=3.0) -> (x < y?=w1021:bool)
                                n718 = Or(x=w1022, y=w1021) -> (x .or. y?=w1020:bool)
                                }
                                }
                                n719 = Index Array(array=w996, index=3) -> (element=w1003:dbl)
                                n720 = global read "rio_Global.vi" "K"() -> (w1011:T11)
                                n721 = global read "rio_Global.vi" "H"() -> (w1010:T11)
                                n722 = global read "rio_Global.vi" "Pp"() -> (w1008:T11)
                                n723 = call-poly <vilib>:"Multiply.vi"("Real Matrix B"=w1010, "Real Matrix A"=w1011) -> ("A * B"=w1009:T11)
                                n724 = global read "rio_Global.vi" "Pp"() -> (w1006:T11)
                                n725 = call-poly <vilib>:"Multiply.vi"("Real Matrix B"=w1008, "Real Matrix A"=w1009) -> ("A * B"=w1007:T11)
                                n726 = call-poly <vilib>:"Subtract.vi"("Real Matrix B"=w1007, "Real Matrix A"=w1006) -> ("A - B"=w1005:T11)
                                n727 = global write "rio_Global.vi" "P"(w1005) -> ()
                                n728 = case shown="True" w999 {
                                tunnel: w1003 -> [w1061 w1068]
                                tunnel: [w1061 w1063] -> w997
                                frame False {
                                }
                                frame True {
                                n729 = global read "rio_Global.vi" "K"() -> (w1067:T11)
                                n730 = Index Array(array=w1067, index (row)=3, index (col)=2 ("disabled index (col)")) -> (element=w1064:dbl)
                                n731 = local read "h_gps"() -> (w1062:dbl)
                                n732 = call "headingweightsum2.vi"("a"=w1064, "h2"=w1062, "h1"=w1068) -> ("a*h2+(1-a)*h1"=w1063:dbl)  [unwired: 8 in]
                                }
                                }
                                n733 = case shown="True" w998 {
                                tunnel: w996 -> [w1037 w1049]
                                tunnel: [w1037 w1048] -> w1002
                                tunnel: w997 -> [_ w1038]
                                frame False {
                                }
                                frame True {
                                n734 = disable-structure shown="Enabled" {
                                disable-tunnel: [w1059 w1060] -> w1039
                                disable-tunnel: w1038 -> [_ w1060]
                                frame Disabled {
                                n735 = local read "h_gps"() -> (w1059:dbl)
                                }
                                frame Enabled {
                                }
                                }
                                n736 = local read "pos_gps"() -> (w1043:dbl[])
                                n737 = call-poly <vilib>:"Array To Matrix.vi"("Real 1D Array"=w1049) -> ("Real Matrix (Column Vector)"=w1053:T11)
                                n738 = Array Subset(array=w1043, index=2, length=2) -> (w1044:dbl[])
                                n739 = Build Array (concatenate)(w1044, w1039) -> (w1040:dbl[])
                                n740 = global read "rio_Global.vi" "H"() -> (w1058:T11)
                                n741 = call-poly <vilib>:"Multiply.vi"("Real Matrix B"=w1053, "Real Matrix A"=w1058) -> ("A * B"=w1057:T11)
                                n742 = call-poly <vilib>:"Array To Matrix.vi"("Real 1D Array"=w1040) -> ("Real Matrix (Column Vector)"=w1056:T11)
                                n743 = call-poly <vilib>:"Subtract.vi"("Real Matrix B"=w1057, "Real Matrix A"=w1056) -> ("A - B"=w1054:T11)
                                n744 = global read "rio_Global.vi" "K"() -> (w1055:T11)
                                n745 = call-poly <vilib>:"Multiply.vi"("Real Matrix B"=w1054, "Real Matrix A"=w1055) -> ("A * B"=w1047:T11)
                                n746 = call-poly <vilib>:"Multiply.vi"("Real Matrix A"=w1047, "Real Scalar c"=0.25) -> ("c * A"=w1045:T11)
                                n747 = call-poly <vilib>:"Add.vi"("Real Matrix B"=w1053, "Real Matrix A"=w1045) -> ("A + B"=w1052:T11)
                                n748 = call-poly <vilib>:"Matrix To Array.vi"("Real Matrix"=w1052) -> ("Real 2D Array"=w1051:dbl[][])
                                n749 = Index Array(array=w1051, index (col)=0 ("disabled index (col)")) -> (element=w1048:dbl[])  [unwired: 1 in]
                                }
                                }
                                n750 = Replace Array Subset(array=w1002, new element=w997, index=3) -> (w1000:dbl[])
                              }
                            }
                          }
                        }
                      }
                    }
                  }
                }
              }
            }
          }
          frame #2 {
            n751 = local read "h_gps"() -> (w1074:dbl)
            n752 = local read "dt"() -> (w1071:dbl)
            n753 = Index Array(array=w1085, index=3) -> (element=w1078:dbl)
            n754 = Array Subset(array=w1085, index=0, length=2) -> (→"pos":dbl[])
            n755 = Greater Than 0?(x=w1071) -> (x > 0?=w1070:bool)
            n756 = call "angleconv.vi"("rad"=w1078) -> ("deg"=→"Heading":dbl)  [unwired: 9 in, 1 out]
            n757 = Greater?(x=1.0, y=w1071) -> (0:w1073:bool)
            n758 = call "headingoperater.vi"("h1"=0.0, "h2"=w1074) -> ("h2+h1"=w1075:dbl)  [unwired: 8 in, 1 out]
            n759 = call "angleconv.vi"("rad"=w1075) -> ("deg"=→"H_GPS":dbl)  [unwired: 9 in, 1 out]
            n760 = Compound Arithmetic op=AND(w1073, w1070) -> (w1069:bool)
            n761 = case shown="True" w1069 {
              tunnel: w1085 -> [_ w1086]
              frame False {
              }
              frame True {
                n762 = flat-sequence {
                  tunnel: w1086 -> [w1110]
                  frame #0 {
                    n763 = Get Date/Time In Seconds() -> (seconds since 1Jan1904=w1101:timestamp)
                    n764 = To Double Precision Float(number=w1101) -> (double precision float=w1095:dbl)
                    n765 = global read "rio_Global.vi" "LCM_POS_T"() -> (w1109:T12)
                    n766 = local read "POS init"() -> (w1091:bool)
                    n767 = Unbundle By Name(w1109) -> ("hash"=w1106:i64)
                    n768 = local read "dt"() -> (w1090:dbl)
                    n769 = Multiply(x=w1095, y=1000000.0) -> (x*y=w1093:dbl)
                    n770 = Array To Cluster(array=w1110) -> (cluster=w1108:T13)
                    n771 = Select(t=0.0, s=w1091, f=w1090) -> (s? t:f=w1088:dbl)
                    n772 = call "hash.vi"("input"=w1106) -> ("output"=w1105:i64)  [unwired: 10 in]
                    n773 = To Quad Integer(1:w1093) -> (0:w1092:i64)
                    n774 = Unbundle(w1108) -> ("Real 2D Array[0]"=w1100:dbl, "Real 2D Array[1]"=w1099:dbl, "Real 2D Array[2]"=w1098:dbl, "Real 2D Array[3]"=w1097:dbl, "Real 2D Array[4]"=w1096:dbl)
                    n775 = Bundle(cluster=w1109, "hash"=w1105, "sys time"=w1092, "dt"=w1088, "x"=w1100, "y"=w1099, "speed"=w1098, "heading"=w1097, "yaw_rate"=w1096) -> (w1087:T12)
                    n776 = Flatten To String(anything=w1087, prepend array or string size? (T)=FALSE) -> (data string=w1103:string)  [unwired: 2 in, 2 out]
                    n777 = global read "rio_Global.vi" "LCM"() -> (w1102:T2)
                    n778 = call "LCM_send.vi"("DATA"=w1103, "ID"="POS_T", "LCM"=w1102) -> ()  [unwired: 6 in, 3 out]
                  }
                }
              }
            }
          }
        }
      }
    }
  }
